vi "Autonomous Independent.vi"() -> ()   [LabVIEW 2016]
doc: "This VI is called when autonomous begins, and will automatically be terminated when autonomous ends. You can carry out timed or sensor driven robot movement independently without needing to return to the caller."
uses:
  <vilib>/Rock Robotics/WPI/ThirdParty/CanMotor/TalonSRX/WPI_CANTalonSRX_APIFeedbackSelect.ctl
  <vilib>/Rock Robotics/WPI/ThirdParty/CanMotor/TalonSRX/WPI_CANTalonSRX_Params.ctl
  <vilib>/Rock Robotics/WPI/ThirdParty/CanMotor/TalonSRX/WPI_CANTalonSRX_APIControlMode.ctl
  <vilib>/Rock Robotics/WPI/Utilities/WPI_GetSetVariantRefNum.vi
  <vilib>/Rock Robotics/Network Tables/NT Read String.vi
  <vilib>/Rock Robotics/Network Tables/NT Write Numeric Array.vi
  <vilib>/Rock Robotics/WPI/RobotDrive/WPI_RobotDriveArcadeDrive_Standard(NoSaturation).vi
  Robot Global Data.vi
panel:
  out "Distance":dbl
  out "RIGHT SIDE":dbl
  out "Encoder Position 4":dbl
  out "Encoder Position 3":dbl
  out "Encoder Position":dbl
  out "Encoder Position 2":dbl
  # "Be sure to right-click and choose Data Operations>>Make Current Value default if you want to save the array values with the VI"
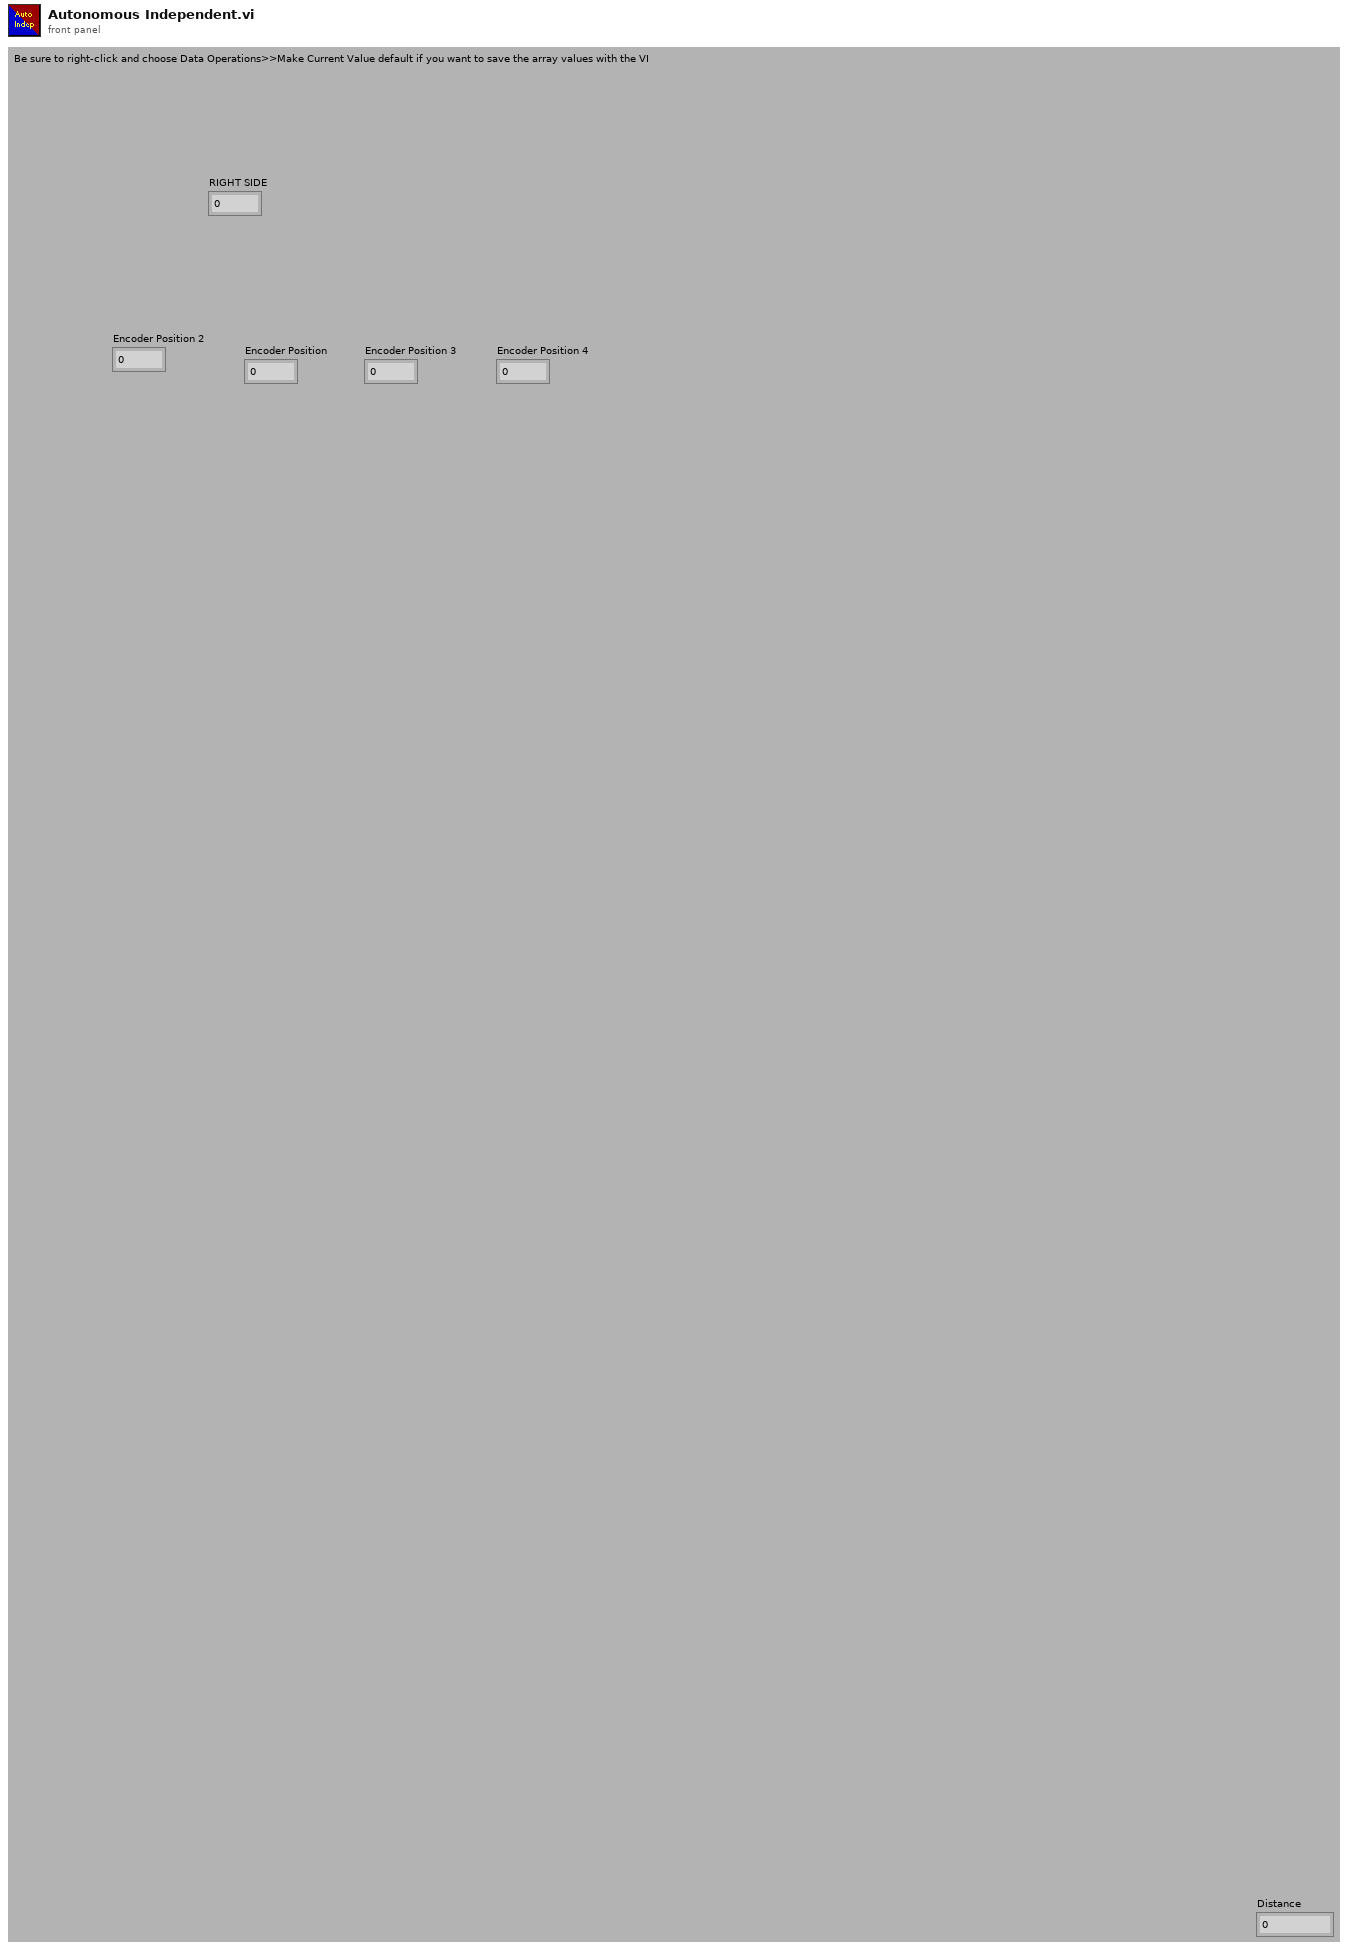
[diagram p1: front panel]
types:
  T1 = typedef "WPI_JoystickDevRef.ctl" = cluster{"Device":T2}
  T2 = typedef "WPI_JoystickDeviceEnum.ctl" = enum16{"USB 0", "USB 1", "USB 2", "USB 3", "USB 4", "USB 5"}
  T3 = typedef "WPI_EncoderDevRef.ctl" = cluster{"DevStatus":errorcluster, "EncoderIndex":T4, "CounterIndex":T5, "DistancePerCount":dbl, "Decoding Type":T6}
  T4 = typedef "FPGA_EncoderIdx.ctl" = enum8{"Enc 0", "Enc 1", "Enc 2", "Enc 3", "Enc 4", "Enc 5", "Enc 6", "Enc 7", "Invalid"}
  T5 = typedef "FPGA_CounterCtrSystemIndex.ctl" = enum8{"Ctr 0", "Ctr 1", "Ctr 2", "Ctr 3", "Ctr 4", "Ctr 5", "Ctr 6", "Ctr 7", "Invalid"}
  T6 = typedef "WPI_EncoderType.ctl" = enum16{"1x", "2x", "4x"}
  T7 = typedef "WPI_MotorControlDeviceRef.ctl" = cluster{"DeviceStatus":errorcluster, "Type":T8, "PWM":cluster{"PWM Channel":T9, "DeadBand":T10}, "CAN":cluster{"Device Number":u8, "SetOutput VI Ref":variant, "GetOutput VI Ref":variant, "Enable VI Ref":variant, "Disable VI Ref":variant, "Data":variant}, "Invert":bool}
  T8 = typedef "WPI_MotorControlType.ctl" = enum16{"PWM", "CAN"}
  T9 = typedef "FPGA_DIOPWMChannel.ctl" = enum8{"PWM 0", "PWM 1", "PWM 2", "PWM 3", "PWM 4", "PWM 5", "PWM 6", "PWM 7", "PWM 8", "PWM 9", "PWM MXP 0", "PWM MXP 1", "PWM MXP 2", "PWM MXP 3", "PWM MXP 4", "PWM MXP 5", "PWM MXP 6", "PWM MXP 7", "PWM MXP 8", "PWM MXP 9", "Invalid"}
  T10 = typedef "WPI_PWMDeadband.ctl" = cluster{"Name":string, "maxPositivePwm":i32, "minPositivePwm":i32, "centerPwm":i32, "maxNegativePwm":i32, "minNegativePwm":i32, "angularRange":u16}
  T11 = typedef "WPI_RobotDriveDevRef.ctl" = cluster{"DevStatus":errorcluster, "Motors[]":T7[], "Square Inputs":bool, "Max Output":dbl}
  T12 = typedef "WPI_CANTalonSRX_APIFeedbackSelect.ctl" = enum16{"Digital Quadrature Encoder", "Analog Potentiometer", "Analog Encoder", "Count on Quad-A (Rising-Edge)", "Count on Quad-A (Falling-Edge)", "CTR Magnetic Enc (Absolute)", "CTR Magnetic Enc (Relative)", "Pulse Width"}
  T13 = typedef "WPI_CANTalonSRX_APIControlMode.ctl" = enum8{"Percent VBus", "Speed", "Position", "Slave", "Unchanged / Invalid", "Voltage Compensation", "Current", "Motion Profile", "Motion Magic"}
  T14 = typedef "WPI_CANTalonSRX_Params.ctl" = u8
  T15 = typedef "WPI_CANTalonSRX_GlobalStatus.ctl" = cluster{"Applied Throttle":dbl, "Module Enabled":bool, "CAN Error":errorcluster, "Closed Loop Error":dbl, "Forward Limit Switch Closed":bool, "Reverse Limit Switch Closed":bool, "Sensor Position":dbl, "Sensor Velocity":dbl, "Current":dbl, "Sticky Fault - Over Temp":bool, "Sticky Fault - Under Voltage":bool, "Sticky Fault - Forward Limit":bool, "Sticky Fault - Reverse Limit":bool, "Sticky Fault - Forward Soft Limit":bool, "Sticky Fault - Reverse Soft Limit":bool, "Brake is Enabled":bool, "Encoder Position":dbl, "Encoder Velocity":dbl, "Encoder Index Count":dbl, "Encoder A Pin State":bool, "Encoder B Pin State":bool, "Encoder Index Pin State":bool, "Analog In":dbl, "Analog In Velocity":dbl, "Temperature (C)":dbl, "Battery Voltage":dbl, "Control 5 Is Supported":bool, "Current Profile Slot Select":dbl, "Pos Div 8":bool, "Vel Div 4":bool, "Pulse Width Position":i32, "Pulse Width Velocity":i32, "Pulse Width Rise To Rise (us)":i32, "Pulse Width Rise To Fall (us)":i32, "Mot Prof Active Is Under Run":bool, "Mot Prof Active Has Under Run":bool, "Mot Prof Active Is Last":bool, "Mot Prof Active Velocity Only":bool, "Mot Prof Active Is Valid":bool, "Mot Prof Buffer Is Full":bool, "Mot Prof Active Profile Slot Select":i32, "Mot Prof NextID":i32, "Mot Prof Count":i32, "Mot Prof Active Velocity":dbl, "Mot Prof Active Position":dbl, "Mot Prof Output Enable":i32, "UsageFrame":u32}
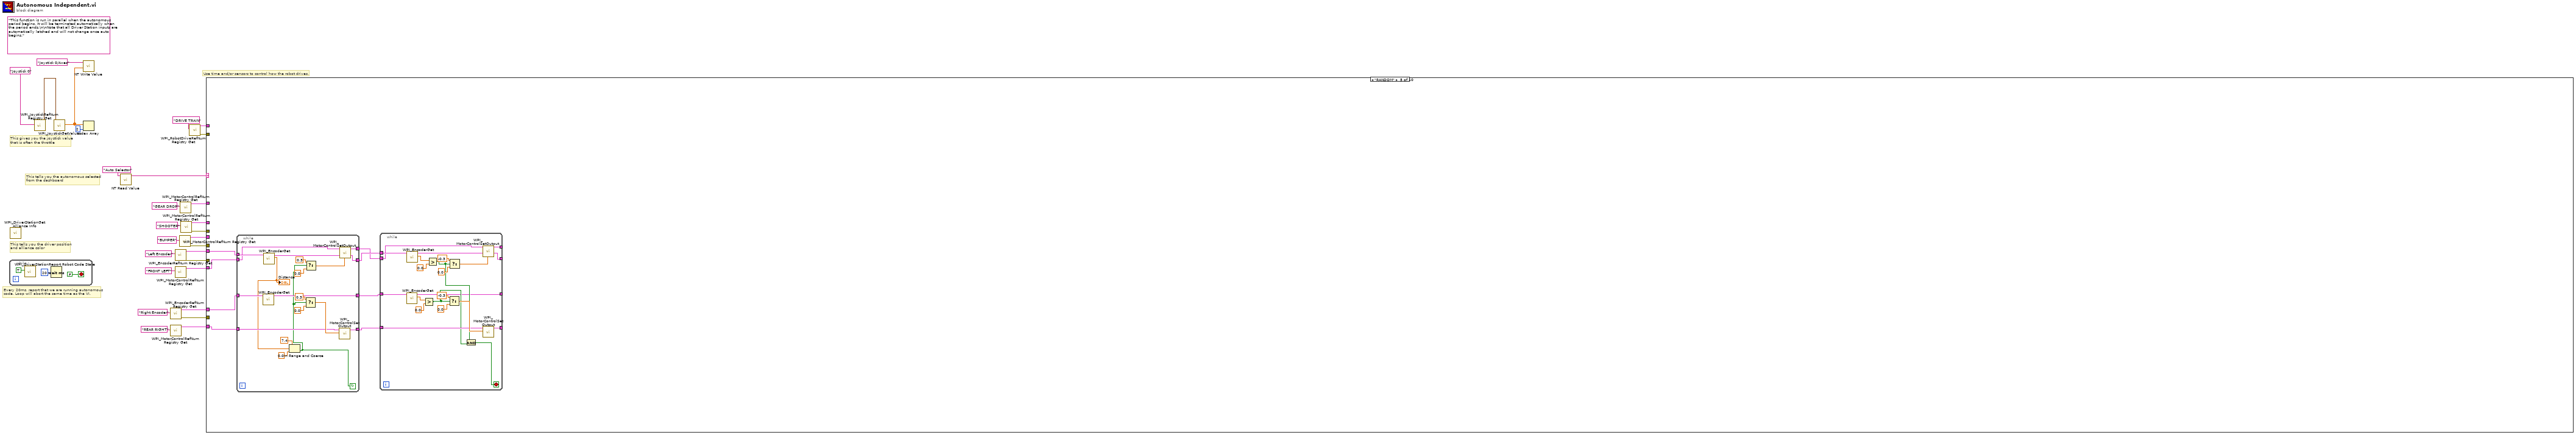
[diagram p0: block diagram]
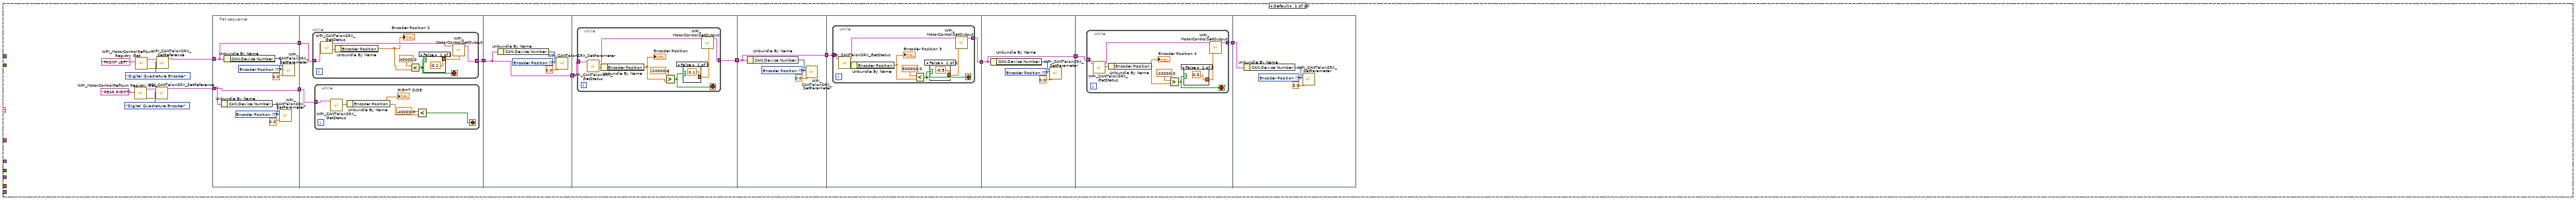
[diagram p2: hidden frame]
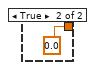
[diagram p3: hidden frame]
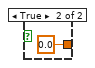
[diagram p4: hidden frame]
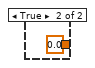
[diagram p5: hidden frame]
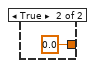
[diagram p6: hidden frame]
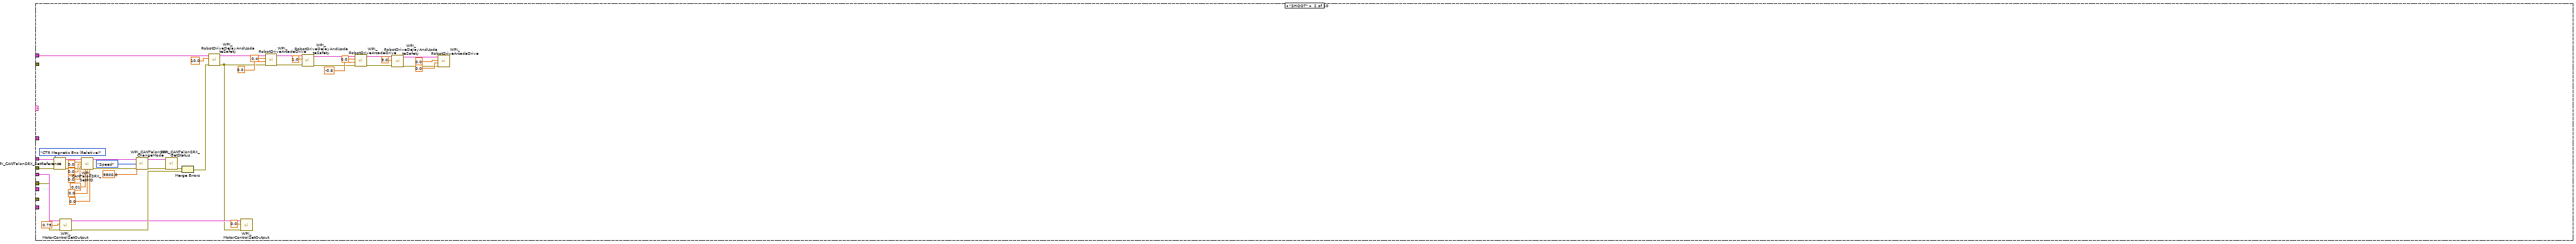
[diagram p7: hidden frame]
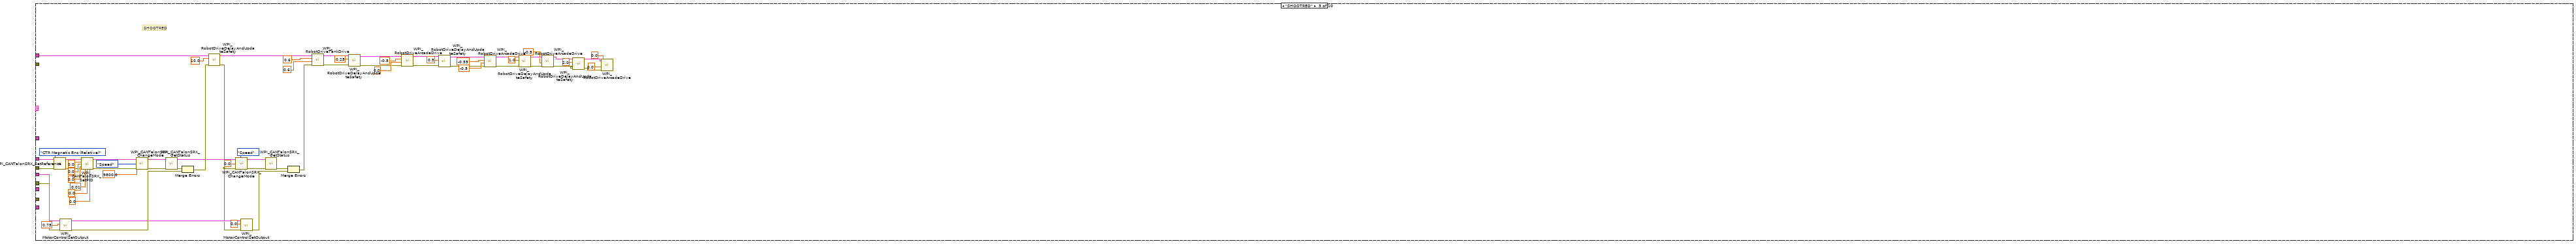
[diagram p8: hidden frame]
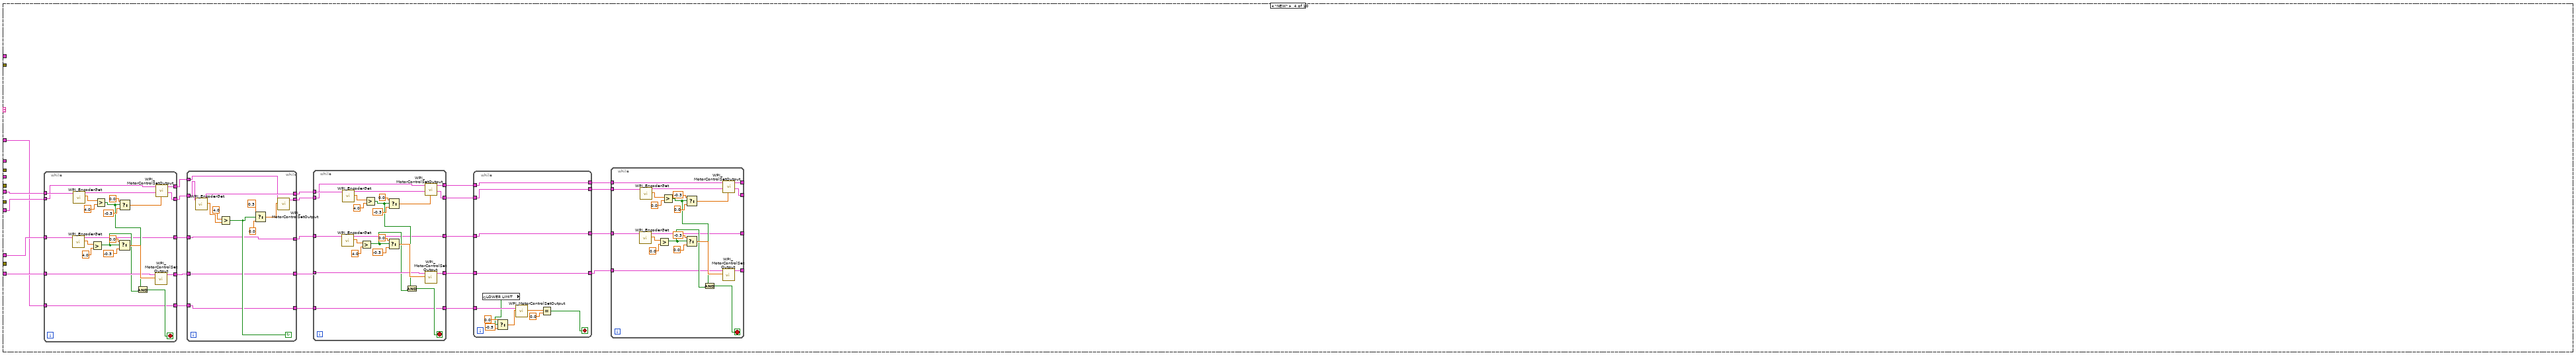
[diagram p9: hidden frame]
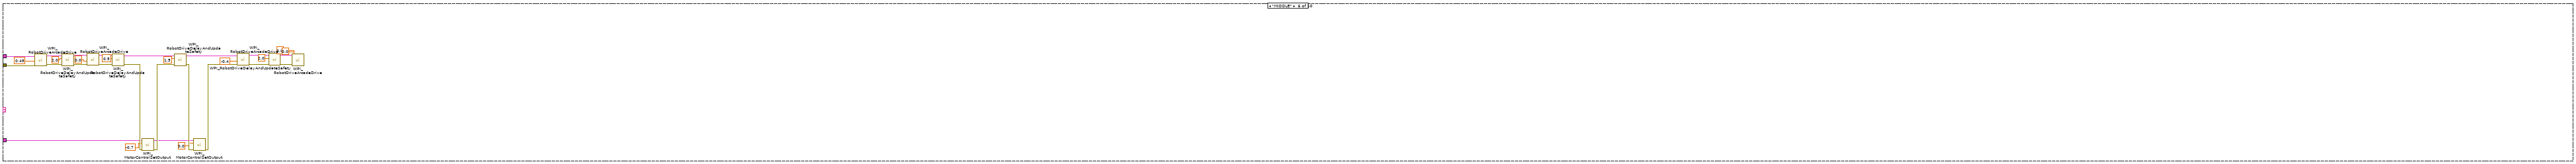
[diagram p10: hidden frame]
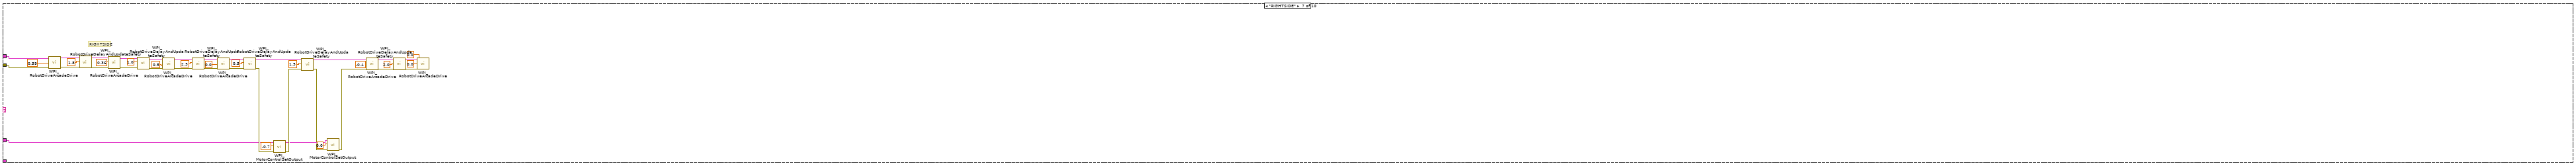
[diagram p11: hidden frame]
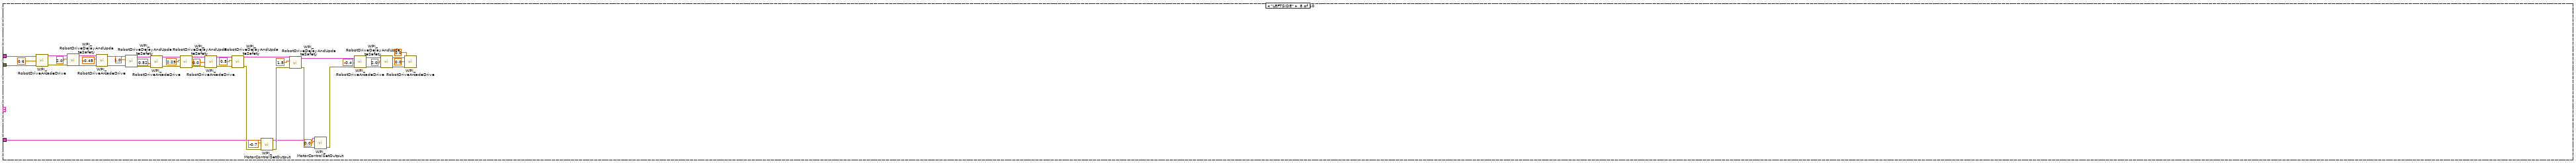
[diagram p12: hidden frame]
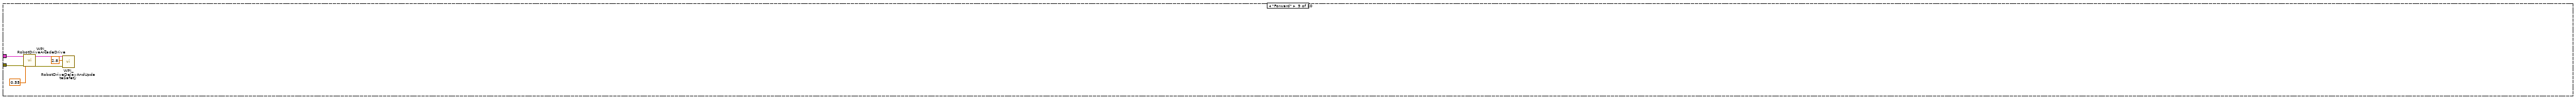
[diagram p13: hidden frame]
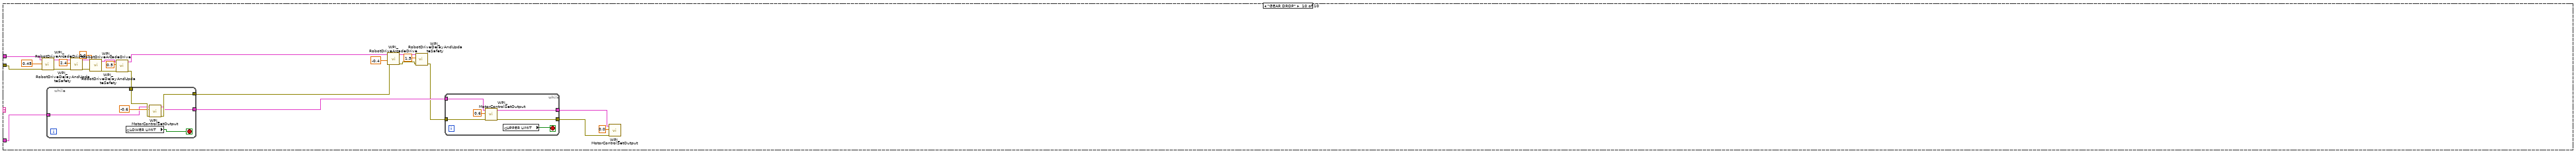
[diagram p14: hidden frame]
diagram:
  (unwired) "This function is run in parallel when the autonomous period begins. It will be terminated automatically when the period ends.\n\nNote that all Driver Station inputs are automatically latched and will not change once auto begins."
  # "Use time and/or sensors to control how the robot drives."
  # "This tells you the autonomous selected\nfrom the dashboard"
  # "Every 20ms, report that we are running autonomous\ncode. Loop will abort the same time as the VI."
  # "This gives you the joystick value\nthat is often the throttle"
  # "This tells you the driver position\nand alliance color"
  n1 = while {
    stop <- FALSE stop-if-true
    n2 = call <vilib>:"WPI_DriverStationReport Robot Code State.vi"("Autonomous"=TRUE) -> ()  [unwired: 10 in, 1 out]
    n3 = Wait (ms)(milliseconds to wait=u32 20) -> ()  [unwired: 1 out]
  }
  n4 = call <vilib>:"WPI_DriverStationGet Alliance Info.vi"() -> ()  [unwired: 12 out]
  n5 = call <vilib>:"WPI_JoystickRefNum Registry Get.vi"("refnum name"="Joystick 0") -> ("JoystickDevRef"=w27:T1)  [unwired: 1 in, 9 out]
  n6 = call <vilib>:"WPI_JoystickGetValues.vi"("JoystickDevRef"=w27) -> ("Axes"=w23:dbl[])  [unwired: 6 in, 4 out]
  n7 = call-poly <vilib>:"NT Write Value.vi"("Numeric Array"=w23, "Name"="Joystick 0/Axes") -> ()  [unwired: 9 in, 1 out]
  n8 = Index Array(array=w23, index=2) -> ()  [unwired: 1 out]
  n9 = call-poly <vilib>:"NT Read Value.vi"("Name"="Auto Selector") -> ("String"=w24:string)  [unwired: 9 in, 1 out]
  n10 = call <vilib>:"WPI_EncoderRefNum Registry Get.vi"("refnum name"="Right Encoder") -> ("error out"=w1:errorcluster, "EncoderDevRef"=w2:T3)  [unwired: 9 in]
  n11 = call <vilib>:"WPI_MotorControlRefNum Registry Get.vi"("refnum name"="REAR RIGHT") -> ("MotorControlDevRef"=w5:T7)  [unwired: 9 in, 1 out]
  n12 = call <vilib>:"WPI_EncoderRefNum Registry Get.vi"("refnum name"="Left Encoder") -> ("error out"=w3:errorcluster, "EncoderDevRef"=w4:T3)  [unwired: 9 in]
  n13 = call <vilib>:"WPI_MotorControlRefNum Registry Get.vi"("refnum name"="FRONT LEFT") -> ("MotorControlDevRef"=w8:T7)  [unwired: 9 in, 1 out]
  n14 = call <vilib>:"WPI_MotorControlRefNum Registry Get.vi"("refnum name"="BUMPER") -> ("error out"=w12:errorcluster, "MotorControlDevRef"=w13:T7)  [unwired: 9 in]
  n15 = call <vilib>:"WPI_MotorControlRefNum Registry Get.vi"("refnum name"="GEAR DROP") -> ("MotorControlDevRef"=w17:T7)  [unwired: 9 in, 1 out]
  n16 = call <vilib>:"WPI_MotorControlRefNum Registry Get.vi"("refnum name"="SHOOTER") -> ("error out"=w14:errorcluster, "MotorControlDevRef"=w15:T7)  [unwired: 9 in]
  n17 = call <vilib>:"WPI_RobotDriveRefNum Registry Get.vi"("refnum name"="DRIVE TRAIN") -> ("error out"=w19:errorcluster, "RobotDriveDevRef"=w20:T11)  [unwired: 9 in]
  n18 = case shown="\"RANDOM\"" w24 {
    tunnel: w20 -> [_ w155 w221 _ _ w431 w434 w517 w523 w548]
    tunnel: w19 -> [_ _ _ _ _ w430 w433 w516 w522 w547]
    tunnel: w17 -> [_ _ _ w247 _ w418 w432 w493 _ w528]
    tunnel: w15 -> [_ w161 w227 _ _ _ _ _ _ _]
    tunnel: w14 -> [_ w160 w226 _ _ _ _ _ _ _]
    tunnel: w13 -> [_ w146 w214 _ _ _ _ _ _ _]
    tunnel: w12 -> [_ w145 w213 _ _ _ _ _ _ _]
    tunnel: w4 -> [_ _ _ w261 w360 _ _ _ _ _]
    tunnel: w8 -> [_ _ _ w260 w361 _ _ _ _ _]
    tunnel: w5 -> [_ _ _ w258 w358 _ _ _ _ _]
    tunnel: w2 -> [_ _ _ w259 w359 _ _ _ _ _]
    tunnel: w3 -> [_ _ _ _ _ _ _ _ _ _]
    tunnel: w1 -> [_ _ _ _ _ _ _ _ _ _]
    frame Default {
      n19 = call <vilib>:"WPI_MotorControlRefNum Registry Get.vi"("refnum name"="REAR RIGHT") -> ("error out"=w36:errorcluster, "MotorControlDevRef"=w35:T7)  [unwired: 9 in]
      n20 = call <vilib>:"WPI_MotorControlRefNum Registry Get.vi"("refnum name"="FRONT LEFT") -> ("error out"=w48:errorcluster, "MotorControlDevRef"=w49:T7)  [unwired: 9 in]
      n21 = call <vilib>:"WPI_CANTalonSRX_SetReference.vi"("error in (no error)"=w36, "Feedback Reference"=WPI_CANTalonSRX_APIFeedbackSelect."Digital Quadrature Encoder", "CAN Talon SRX Ref"=w35) -> ("CAN Talon SRX Ref"=w33:T7)  [unwired: 7 in, 1 out]
      n22 = call <vilib>:"WPI_CANTalonSRX_SetReference.vi"("error in (no error)"=w48, "Feedback Reference"=WPI_CANTalonSRX_APIFeedbackSelect."Digital Quadrature Encoder", "CAN Talon SRX Ref"=w49) -> ("CAN Talon SRX Ref"=w44:T7)  [unwired: 7 in, 1 out]
      n23 = flat-sequence {
        tunnel: w44 -> [w55]
        tunnel: [w55] -> w43
        tunnel: w33 -> [w51]
        tunnel: [w51] -> w32
        tunnel: [w60] -> w46
        tunnel: w43 -> [w61]
        tunnel: w32 -> [w59]
        tunnel: w46 -> [w77]
        tunnel: [w77] -> w45
        tunnel: w45 -> [w82]
        tunnel: [w81] -> w42
        tunnel: w42 -> [w93]
        tunnel: [w93] -> w41
        tunnel: w41 -> [w98]
        tunnel: [w97] -> w40
        tunnel: w40 -> [w109]
        tunnel: [w109] -> w39
        tunnel: w39 -> [w114]
        tunnel: [w113] -> w38
        tunnel: w38 -> [w125]
        frame #0 {
          w53 = T14 77 items=["Slot 0 - P"=1, "Slot 0 - I"=2, "Slot 0 - D"=3, "Slot 0 - F"=4, "Slot 0 - I Zone"=5, "Slot 0 - Ramp Rate"=6, "Slot 1 - P"=11, "Slot 1 - I"=12, "Slot 1 - D"=13, "Slot 1 - F"=14, "Slot 1 - I Zone"=15, "Slot 1 - Ramp Rate"=16, "Soft Limit - Forward"=21, "Soft Limit - Reverse"=22, "Soft Limit - Forward Enable"=23, "Soft Limit - Reverse Enable"=24, "On Boot - Brake Mode"=31, "On Boot - Limit Normally Closed - Forward"=32, "On Boot - Limit Normally Closed - Reverse"=33, "On Boot - Limit Disabled - Forward"=34, "On Boot - Limit Disabled - Reverse"=35, "Fault - Over Temp"=41, "Fault - Under Voltage"=42, "Fault - Forward Limit"=43, "Fault - Reverse Limit"=44, "Fault - Hardware Failure"=45, "Fault - Forward Soft Limit"=46, "Fault - Reverse Soft Limit"=47, "Sticky Fault - Over Temp"=48, "Sticky Fault - Under Voltage"=49, "Sticky Fault - Forward Limit"=50, "Sticky Fault - Reverse Limit"=51, "Sticky Fault - Forward Soft Limit"=52, "Sticky Fault - Reverse Soft Limit"=53, "Applied Throttle"=61, "Closed-Loop Error"=62, "Select Feedback Device"=63, "Reverse Closed-Loop Output"=64, "Mode Select"=65, "Profile Slot Select"=66, "Ramp Throttle"=67, "Reverse Feedback Sensor"=68, "Limit Switch Enabled"=69, "Limit Switch Closed - Forward"=70, "Limit Switch Closed - Reverse"=71, "Sensor Position"=73, "Sensor Velocity"=74, "Current"=75, "Brake is Enabled"=76, "Encoder Position"=77, "Encoder Velocity"=78, "Encoder Index Rise Events"=79, "Encoder A Pin State"=80, "Encoder B Pin State"=81, "Encoder Index Pin State"=82, "Analog In with Overflow"=83, "Analog In Velocity"=84, "Temperature"=85, "Battery Voltage"=86, "Reset Count"=87, "Reset Flags"=88, "Firmware Version"=89, "Settings Changed"=90, "Quad Filter Enable"=91, "Ignore Disable Broadcast"=92, "I Accumulator"=93, "Status 1 Frame Rate Ms"=94, "Status 2 Frame Rate Ms"=95, "Status 3 Frame Rate Ms"=96, "Status 4 Frame Rate Ms"=97, "Status 6 Frame Rate Ms"=98, "Status 7 Frame Rate Ms"=99, "Enable Index Pin Clear Position"=100, "Peak Positive Output"=104, "Nominal Positive Output"=105, "Peak Negative Output"=106, "Nominal Negative Output"=107, "Quad Index Pin Polarity"=108, "Status 8 Frame Rate Ms"=109, "Allow Position Overflow"=110, "Slot 0 - Allowable Closed-Loop Error"=111, "Number Potentiometer Turns"=112, "Encoder Codes Per Rev"=113, "Pulse Width Decoded Position"=114, "Analog Position"=115, "Voltage Compensation Rate (V/s)"=116, "Slot 1 - Allowable Closed-Loop Error"=117, "Motion Profile Has Underrun Err"=119, "Reserved 120"=120, "Legacy Control Mode"=121, "Motion Magic Acceleration"=122, "Motion Magic Cruise Velocity"=123, "Status 10 Frame Rate"=124, "Current Limit Threshold"=125, "CustomParam0"=137, "CustomParam1"=138, "PersStorageSaving"=139, "ClearPositionOnLimitF"=144, "ClearPositionOnLimitR"=145, "NominalBatteryVoltage"=146, "SampleVelocityPeriod"=147, "SampleVelocityWindow"=148] ("Parameter")
          w57 = T14 77 items=["Slot 0 - P"=1, "Slot 0 - I"=2, "Slot 0 - D"=3, "Slot 0 - F"=4, "Slot 0 - I Zone"=5, "Slot 0 - Ramp Rate"=6, "Slot 1 - P"=11, "Slot 1 - I"=12, "Slot 1 - D"=13, "Slot 1 - F"=14, "Slot 1 - I Zone"=15, "Slot 1 - Ramp Rate"=16, "Soft Limit - Forward"=21, "Soft Limit - Reverse"=22, "Soft Limit - Forward Enable"=23, "Soft Limit - Reverse Enable"=24, "On Boot - Brake Mode"=31, "On Boot - Limit Normally Closed - Forward"=32, "On Boot - Limit Normally Closed - Reverse"=33, "On Boot - Limit Disabled - Forward"=34, "On Boot - Limit Disabled - Reverse"=35, "Fault - Over Temp"=41, "Fault - Under Voltage"=42, "Fault - Forward Limit"=43, "Fault - Reverse Limit"=44, "Fault - Hardware Failure"=45, "Fault - Forward Soft Limit"=46, "Fault - Reverse Soft Limit"=47, "Sticky Fault - Over Temp"=48, "Sticky Fault - Under Voltage"=49, "Sticky Fault - Forward Limit"=50, "Sticky Fault - Reverse Limit"=51, "Sticky Fault - Forward Soft Limit"=52, "Sticky Fault - Reverse Soft Limit"=53, "Applied Throttle"=61, "Closed-Loop Error"=62, "Select Feedback Device"=63, "Reverse Closed-Loop Output"=64, "Mode Select"=65, "Profile Slot Select"=66, "Ramp Throttle"=67, "Reverse Feedback Sensor"=68, "Limit Switch Enabled"=69, "Limit Switch Closed - Forward"=70, "Limit Switch Closed - Reverse"=71, "Sensor Position"=73, "Sensor Velocity"=74, "Current"=75, "Brake is Enabled"=76, "Encoder Position"=77, "Encoder Velocity"=78, "Encoder Index Rise Events"=79, "Encoder A Pin State"=80, "Encoder B Pin State"=81, "Encoder Index Pin State"=82, "Analog In with Overflow"=83, "Analog In Velocity"=84, "Temperature"=85, "Battery Voltage"=86, "Reset Count"=87, "Reset Flags"=88, "Firmware Version"=89, "Settings Changed"=90, "Quad Filter Enable"=91, "Ignore Disable Broadcast"=92, "I Accumulator"=93, "Status 1 Frame Rate Ms"=94, "Status 2 Frame Rate Ms"=95, "Status 3 Frame Rate Ms"=96, "Status 4 Frame Rate Ms"=97, "Status 6 Frame Rate Ms"=98, "Status 7 Frame Rate Ms"=99, "Enable Index Pin Clear Position"=100, "Peak Positive Output"=104, "Nominal Positive Output"=105, "Peak Negative Output"=106, "Nominal Negative Output"=107, "Quad Index Pin Polarity"=108, "Status 8 Frame Rate Ms"=109, "Allow Position Overflow"=110, "Slot 0 - Allowable Closed-Loop Error"=111, "Number Potentiometer Turns"=112, "Encoder Codes Per Rev"=113, "Pulse Width Decoded Position"=114, "Analog Position"=115, "Voltage Compensation Rate (V/s)"=116, "Slot 1 - Allowable Closed-Loop Error"=117, "Motion Profile Has Underrun Err"=119, "Reserved 120"=120, "Legacy Control Mode"=121, "Motion Magic Acceleration"=122, "Motion Magic Cruise Velocity"=123, "Status 10 Frame Rate"=124, "Current Limit Threshold"=125, "CustomParam0"=137, "CustomParam1"=138, "PersStorageSaving"=139, "ClearPositionOnLimitF"=144, "ClearPositionOnLimitR"=145, "NominalBatteryVoltage"=146, "SampleVelocityPeriod"=147, "SampleVelocityWindow"=148] ("Parameter")
          n24 = Unbundle By Name(w51) -> ("CAN.Device Number"=w52:u8)
          n25 = Unbundle By Name(w55) -> ("CAN.Device Number"=w58:u8)
          n26 = call <vilib>:"WPI_CANTalonSRX_SetParameter.vi"("Value"=0.0, "Parameter"=w53, "Device ID (0)"=w52) -> ()  [unwired: 7 in, 2 out]
          n27 = call <vilib>:"WPI_CANTalonSRX_SetParameter.vi"("Value"=0.0, "Parameter"=w57, "Device ID (0)"=w58) -> ()  [unwired: 7 in, 2 out]
        }
        frame #1 {
          n28 = while {
            tunnel: w61 -> [w68]
            tunnel: [w67] -> w60
            stop <- w71 stop-if-true
            n29 = call <vilib>:"WPI_CANTalonSRX_GetStatus.vi"("CAN Talon SRX Ref"=w68) -> ("Talon SRX Status"=w74:T15, "CAN Talon SRX Ref"=w73:T7)  [unwired: 8 in, 1 out]
            n30 = Unbundle By Name(w74) -> ("Encoder Position"=w70:dbl)
            "Encoder Position 2" <- w70
            n31 = Less?(x=40000.0, y=w70) -> (x < y?=w71:bool)
            n32 = case shown="False" w71 {
              tunnel: [-0.1 ("x") 0.0 ("x")] -> w72
              frame False {
              }
              frame True {
              }
            }
            n33 = call <vilib>:"WPI_MotorControlSetOutput.vi"("Output"=w72, "MotorControlDevRef"=w73) -> ("MotorControlDevRef"=w67:T7)  [unwired: 7 in, 2 out]
          }
          n34 = while {
            tunnel: w59 -> [w66]
            stop <- w63 stop-if-true
            n35 = call <vilib>:"WPI_CANTalonSRX_GetStatus.vi"("CAN Talon SRX Ref"=w66) -> ("Talon SRX Status"=w62:T15)  [unwired: 8 in, 2 out]
            n36 = Unbundle By Name(w62) -> ("Encoder Position"=w65:dbl)
            "RIGHT SIDE" <- w65
            n37 = Less?(x=-40000.0, y=w65) -> (x < y?=w63:bool)
          }
        }
        frame #2 {
          w79 = T14 77 items=["Slot 0 - P"=1, "Slot 0 - I"=2, "Slot 0 - D"=3, "Slot 0 - F"=4, "Slot 0 - I Zone"=5, "Slot 0 - Ramp Rate"=6, "Slot 1 - P"=11, "Slot 1 - I"=12, "Slot 1 - D"=13, "Slot 1 - F"=14, "Slot 1 - I Zone"=15, "Slot 1 - Ramp Rate"=16, "Soft Limit - Forward"=21, "Soft Limit - Reverse"=22, "Soft Limit - Forward Enable"=23, "Soft Limit - Reverse Enable"=24, "On Boot - Brake Mode"=31, "On Boot - Limit Normally Closed - Forward"=32, "On Boot - Limit Normally Closed - Reverse"=33, "On Boot - Limit Disabled - Forward"=34, "On Boot - Limit Disabled - Reverse"=35, "Fault - Over Temp"=41, "Fault - Under Voltage"=42, "Fault - Forward Limit"=43, "Fault - Reverse Limit"=44, "Fault - Hardware Failure"=45, "Fault - Forward Soft Limit"=46, "Fault - Reverse Soft Limit"=47, "Sticky Fault - Over Temp"=48, "Sticky Fault - Under Voltage"=49, "Sticky Fault - Forward Limit"=50, "Sticky Fault - Reverse Limit"=51, "Sticky Fault - Forward Soft Limit"=52, "Sticky Fault - Reverse Soft Limit"=53, "Applied Throttle"=61, "Closed-Loop Error"=62, "Select Feedback Device"=63, "Reverse Closed-Loop Output"=64, "Mode Select"=65, "Profile Slot Select"=66, "Ramp Throttle"=67, "Reverse Feedback Sensor"=68, "Limit Switch Enabled"=69, "Limit Switch Closed - Forward"=70, "Limit Switch Closed - Reverse"=71, "Sensor Position"=73, "Sensor Velocity"=74, "Current"=75, "Brake is Enabled"=76, "Encoder Position"=77, "Encoder Velocity"=78, "Encoder Index Rise Events"=79, "Encoder A Pin State"=80, "Encoder B Pin State"=81, "Encoder Index Pin State"=82, "Analog In with Overflow"=83, "Analog In Velocity"=84, "Temperature"=85, "Battery Voltage"=86, "Reset Count"=87, "Reset Flags"=88, "Firmware Version"=89, "Settings Changed"=90, "Quad Filter Enable"=91, "Ignore Disable Broadcast"=92, "I Accumulator"=93, "Status 1 Frame Rate Ms"=94, "Status 2 Frame Rate Ms"=95, "Status 3 Frame Rate Ms"=96, "Status 4 Frame Rate Ms"=97, "Status 6 Frame Rate Ms"=98, "Status 7 Frame Rate Ms"=99, "Enable Index Pin Clear Position"=100, "Peak Positive Output"=104, "Nominal Positive Output"=105, "Peak Negative Output"=106, "Nominal Negative Output"=107, "Quad Index Pin Polarity"=108, "Status 8 Frame Rate Ms"=109, "Allow Position Overflow"=110, "Slot 0 - Allowable Closed-Loop Error"=111, "Number Potentiometer Turns"=112, "Encoder Codes Per Rev"=113, "Pulse Width Decoded Position"=114, "Analog Position"=115, "Voltage Compensation Rate (V/s)"=116, "Slot 1 - Allowable Closed-Loop Error"=117, "Motion Profile Has Underrun Err"=119, "Reserved 120"=120, "Legacy Control Mode"=121, "Motion Magic Acceleration"=122, "Motion Magic Cruise Velocity"=123, "Status 10 Frame Rate"=124, "Current Limit Threshold"=125, "CustomParam0"=137, "CustomParam1"=138, "PersStorageSaving"=139, "ClearPositionOnLimitF"=144, "ClearPositionOnLimitR"=145, "NominalBatteryVoltage"=146, "SampleVelocityPeriod"=147, "SampleVelocityWindow"=148] ("Parameter")
          n38 = Unbundle By Name(w77) -> ("CAN.Device Number"=w80:u8)
          n39 = call <vilib>:"WPI_CANTalonSRX_SetParameter.vi"("Value"=0.0, "Parameter"=w79, "Device ID (0)"=w80) -> ()  [unwired: 7 in, 2 out]
        }
        frame #3 {
          n40 = while {
            tunnel: w82 -> [w84]
            tunnel: [w83] -> w81
            stop <- w87 stop-if-true
            n41 = call <vilib>:"WPI_CANTalonSRX_GetStatus.vi"("CAN Talon SRX Ref"=w84) -> ("Talon SRX Status"=w90:T15, "CAN Talon SRX Ref"=w89:T7)  [unwired: 8 in, 1 out]
            n42 = Unbundle By Name(w90) -> ("Encoder Position"=w86:dbl)
            "Encoder Position" <- w86
            n43 = Greater?(x=-20000.0 ("y"), y=w86) -> (0:w87:bool)
            n44 = case shown="False" w87 {
              tunnel: [0.1 ("x") 0.0 ("x")] -> w88
              frame False {
              }
              frame True {
              }
            }
            n45 = call <vilib>:"WPI_MotorControlSetOutput.vi"("Output"=w88, "MotorControlDevRef"=w89) -> ("MotorControlDevRef"=w83:T7)  [unwired: 7 in, 2 out]
          }
        }
        frame #4 {
          w95 = T14 77 items=["Slot 0 - P"=1, "Slot 0 - I"=2, "Slot 0 - D"=3, "Slot 0 - F"=4, "Slot 0 - I Zone"=5, "Slot 0 - Ramp Rate"=6, "Slot 1 - P"=11, "Slot 1 - I"=12, "Slot 1 - D"=13, "Slot 1 - F"=14, "Slot 1 - I Zone"=15, "Slot 1 - Ramp Rate"=16, "Soft Limit - Forward"=21, "Soft Limit - Reverse"=22, "Soft Limit - Forward Enable"=23, "Soft Limit - Reverse Enable"=24, "On Boot - Brake Mode"=31, "On Boot - Limit Normally Closed - Forward"=32, "On Boot - Limit Normally Closed - Reverse"=33, "On Boot - Limit Disabled - Forward"=34, "On Boot - Limit Disabled - Reverse"=35, "Fault - Over Temp"=41, "Fault - Under Voltage"=42, "Fault - Forward Limit"=43, "Fault - Reverse Limit"=44, "Fault - Hardware Failure"=45, "Fault - Forward Soft Limit"=46, "Fault - Reverse Soft Limit"=47, "Sticky Fault - Over Temp"=48, "Sticky Fault - Under Voltage"=49, "Sticky Fault - Forward Limit"=50, "Sticky Fault - Reverse Limit"=51, "Sticky Fault - Forward Soft Limit"=52, "Sticky Fault - Reverse Soft Limit"=53, "Applied Throttle"=61, "Closed-Loop Error"=62, "Select Feedback Device"=63, "Reverse Closed-Loop Output"=64, "Mode Select"=65, "Profile Slot Select"=66, "Ramp Throttle"=67, "Reverse Feedback Sensor"=68, "Limit Switch Enabled"=69, "Limit Switch Closed - Forward"=70, "Limit Switch Closed - Reverse"=71, "Sensor Position"=73, "Sensor Velocity"=74, "Current"=75, "Brake is Enabled"=76, "Encoder Position"=77, "Encoder Velocity"=78, "Encoder Index Rise Events"=79, "Encoder A Pin State"=80, "Encoder B Pin State"=81, "Encoder Index Pin State"=82, "Analog In with Overflow"=83, "Analog In Velocity"=84, "Temperature"=85, "Battery Voltage"=86, "Reset Count"=87, "Reset Flags"=88, "Firmware Version"=89, "Settings Changed"=90, "Quad Filter Enable"=91, "Ignore Disable Broadcast"=92, "I Accumulator"=93, "Status 1 Frame Rate Ms"=94, "Status 2 Frame Rate Ms"=95, "Status 3 Frame Rate Ms"=96, "Status 4 Frame Rate Ms"=97, "Status 6 Frame Rate Ms"=98, "Status 7 Frame Rate Ms"=99, "Enable Index Pin Clear Position"=100, "Peak Positive Output"=104, "Nominal Positive Output"=105, "Peak Negative Output"=106, "Nominal Negative Output"=107, "Quad Index Pin Polarity"=108, "Status 8 Frame Rate Ms"=109, "Allow Position Overflow"=110, "Slot 0 - Allowable Closed-Loop Error"=111, "Number Potentiometer Turns"=112, "Encoder Codes Per Rev"=113, "Pulse Width Decoded Position"=114, "Analog Position"=115, "Voltage Compensation Rate (V/s)"=116, "Slot 1 - Allowable Closed-Loop Error"=117, "Motion Profile Has Underrun Err"=119, "Reserved 120"=120, "Legacy Control Mode"=121, "Motion Magic Acceleration"=122, "Motion Magic Cruise Velocity"=123, "Status 10 Frame Rate"=124, "Current Limit Threshold"=125, "CustomParam0"=137, "CustomParam1"=138, "PersStorageSaving"=139, "ClearPositionOnLimitF"=144, "ClearPositionOnLimitR"=145, "NominalBatteryVoltage"=146, "SampleVelocityPeriod"=147, "SampleVelocityWindow"=148] ("Parameter")
          n46 = Unbundle By Name(w93) -> ("CAN.Device Number"=w96:u8)
          n47 = call <vilib>:"WPI_CANTalonSRX_SetParameter.vi"("Value"=0.0, "Parameter"=w95, "Device ID (0)"=w96) -> ()  [unwired: 7 in, 2 out]
        }
        frame #5 {
          n48 = while {
            tunnel: w98 -> [w100]
            tunnel: [w99] -> w97
            stop <- w103 stop-if-true
            n49 = call <vilib>:"WPI_CANTalonSRX_GetStatus.vi"("CAN Talon SRX Ref"=w100) -> ("Talon SRX Status"=w106:T15, "CAN Talon SRX Ref"=w105:T7)  [unwired: 8 in, 1 out]
            n50 = Unbundle By Name(w106) -> ("Encoder Position"=w102:dbl)
            "Encoder Position 3" <- w102
            n51 = Less?(x=500000.0, y=w102) -> (x < y?=w103:bool)
            n52 = case shown="False" w103 {
              tunnel: [-0.5 ("x") 0.0 ("x")] -> w104
              frame False {
              }
              frame True {
              }
            }
            n53 = call <vilib>:"WPI_MotorControlSetOutput.vi"("Output"=w104, "MotorControlDevRef"=w105) -> ("MotorControlDevRef"=w99:T7)  [unwired: 7 in, 2 out]
          }
        }
        frame #6 {
          w111 = T14 77 items=["Slot 0 - P"=1, "Slot 0 - I"=2, "Slot 0 - D"=3, "Slot 0 - F"=4, "Slot 0 - I Zone"=5, "Slot 0 - Ramp Rate"=6, "Slot 1 - P"=11, "Slot 1 - I"=12, "Slot 1 - D"=13, "Slot 1 - F"=14, "Slot 1 - I Zone"=15, "Slot 1 - Ramp Rate"=16, "Soft Limit - Forward"=21, "Soft Limit - Reverse"=22, "Soft Limit - Forward Enable"=23, "Soft Limit - Reverse Enable"=24, "On Boot - Brake Mode"=31, "On Boot - Limit Normally Closed - Forward"=32, "On Boot - Limit Normally Closed - Reverse"=33, "On Boot - Limit Disabled - Forward"=34, "On Boot - Limit Disabled - Reverse"=35, "Fault - Over Temp"=41, "Fault - Under Voltage"=42, "Fault - Forward Limit"=43, "Fault - Reverse Limit"=44, "Fault - Hardware Failure"=45, "Fault - Forward Soft Limit"=46, "Fault - Reverse Soft Limit"=47, "Sticky Fault - Over Temp"=48, "Sticky Fault - Under Voltage"=49, "Sticky Fault - Forward Limit"=50, "Sticky Fault - Reverse Limit"=51, "Sticky Fault - Forward Soft Limit"=52, "Sticky Fault - Reverse Soft Limit"=53, "Applied Throttle"=61, "Closed-Loop Error"=62, "Select Feedback Device"=63, "Reverse Closed-Loop Output"=64, "Mode Select"=65, "Profile Slot Select"=66, "Ramp Throttle"=67, "Reverse Feedback Sensor"=68, "Limit Switch Enabled"=69, "Limit Switch Closed - Forward"=70, "Limit Switch Closed - Reverse"=71, "Sensor Position"=73, "Sensor Velocity"=74, "Current"=75, "Brake is Enabled"=76, "Encoder Position"=77, "Encoder Velocity"=78, "Encoder Index Rise Events"=79, "Encoder A Pin State"=80, "Encoder B Pin State"=81, "Encoder Index Pin State"=82, "Analog In with Overflow"=83, "Analog In Velocity"=84, "Temperature"=85, "Battery Voltage"=86, "Reset Count"=87, "Reset Flags"=88, "Firmware Version"=89, "Settings Changed"=90, "Quad Filter Enable"=91, "Ignore Disable Broadcast"=92, "I Accumulator"=93, "Status 1 Frame Rate Ms"=94, "Status 2 Frame Rate Ms"=95, "Status 3 Frame Rate Ms"=96, "Status 4 Frame Rate Ms"=97, "Status 6 Frame Rate Ms"=98, "Status 7 Frame Rate Ms"=99, "Enable Index Pin Clear Position"=100, "Peak Positive Output"=104, "Nominal Positive Output"=105, "Peak Negative Output"=106, "Nominal Negative Output"=107, "Quad Index Pin Polarity"=108, "Status 8 Frame Rate Ms"=109, "Allow Position Overflow"=110, "Slot 0 - Allowable Closed-Loop Error"=111, "Number Potentiometer Turns"=112, "Encoder Codes Per Rev"=113, "Pulse Width Decoded Position"=114, "Analog Position"=115, "Voltage Compensation Rate (V/s)"=116, "Slot 1 - Allowable Closed-Loop Error"=117, "Motion Profile Has Underrun Err"=119, "Reserved 120"=120, "Legacy Control Mode"=121, "Motion Magic Acceleration"=122, "Motion Magic Cruise Velocity"=123, "Status 10 Frame Rate"=124, "Current Limit Threshold"=125, "CustomParam0"=137, "CustomParam1"=138, "PersStorageSaving"=139, "ClearPositionOnLimitF"=144, "ClearPositionOnLimitR"=145, "NominalBatteryVoltage"=146, "SampleVelocityPeriod"=147, "SampleVelocityWindow"=148] ("Parameter")
          n54 = Unbundle By Name(w109) -> ("CAN.Device Number"=w110:u8)
          n55 = call <vilib>:"WPI_CANTalonSRX_SetParameter.vi"("Value"=0.0, "Parameter"=w111, "Device ID (0)"=w110) -> ()  [unwired: 7 in, 2 out]
        }
        frame #7 {
          n56 = while {
            tunnel: w114 -> [w116]
            tunnel: [w115] -> w113
            stop <- w119 stop-if-true
            n57 = call <vilib>:"WPI_CANTalonSRX_GetStatus.vi"("CAN Talon SRX Ref"=w116) -> ("Talon SRX Status"=w122:T15, "CAN Talon SRX Ref"=w121:T7)  [unwired: 8 in, 1 out]
            n58 = Unbundle By Name(w122) -> ("Encoder Position"=w118:dbl)
            "Encoder Position 4" <- w118
            n59 = Greater?(x=-20000.0, y=w118) -> (0:w119:bool)
            n60 = case shown="False" w119 {
              tunnel: [0.3 ("x") 0.0 ("x")] -> w120
              frame False {
              }
              frame True {
              }
            }
            n61 = call <vilib>:"WPI_MotorControlSetOutput.vi"("Output"=w120, "MotorControlDevRef"=w121) -> ("MotorControlDevRef"=w115:T7)  [unwired: 7 in, 2 out]
          }
        }
        frame #8 {
          w127 = T14 77 items=["Slot 0 - P"=1, "Slot 0 - I"=2, "Slot 0 - D"=3, "Slot 0 - F"=4, "Slot 0 - I Zone"=5, "Slot 0 - Ramp Rate"=6, "Slot 1 - P"=11, "Slot 1 - I"=12, "Slot 1 - D"=13, "Slot 1 - F"=14, "Slot 1 - I Zone"=15, "Slot 1 - Ramp Rate"=16, "Soft Limit - Forward"=21, "Soft Limit - Reverse"=22, "Soft Limit - Forward Enable"=23, "Soft Limit - Reverse Enable"=24, "On Boot - Brake Mode"=31, "On Boot - Limit Normally Closed - Forward"=32, "On Boot - Limit Normally Closed - Reverse"=33, "On Boot - Limit Disabled - Forward"=34, "On Boot - Limit Disabled - Reverse"=35, "Fault - Over Temp"=41, "Fault - Under Voltage"=42, "Fault - Forward Limit"=43, "Fault - Reverse Limit"=44, "Fault - Hardware Failure"=45, "Fault - Forward Soft Limit"=46, "Fault - Reverse Soft Limit"=47, "Sticky Fault - Over Temp"=48, "Sticky Fault - Under Voltage"=49, "Sticky Fault - Forward Limit"=50, "Sticky Fault - Reverse Limit"=51, "Sticky Fault - Forward Soft Limit"=52, "Sticky Fault - Reverse Soft Limit"=53, "Applied Throttle"=61, "Closed-Loop Error"=62, "Select Feedback Device"=63, "Reverse Closed-Loop Output"=64, "Mode Select"=65, "Profile Slot Select"=66, "Ramp Throttle"=67, "Reverse Feedback Sensor"=68, "Limit Switch Enabled"=69, "Limit Switch Closed - Forward"=70, "Limit Switch Closed - Reverse"=71, "Sensor Position"=73, "Sensor Velocity"=74, "Current"=75, "Brake is Enabled"=76, "Encoder Position"=77, "Encoder Velocity"=78, "Encoder Index Rise Events"=79, "Encoder A Pin State"=80, "Encoder B Pin State"=81, "Encoder Index Pin State"=82, "Analog In with Overflow"=83, "Analog In Velocity"=84, "Temperature"=85, "Battery Voltage"=86, "Reset Count"=87, "Reset Flags"=88, "Firmware Version"=89, "Settings Changed"=90, "Quad Filter Enable"=91, "Ignore Disable Broadcast"=92, "I Accumulator"=93, "Status 1 Frame Rate Ms"=94, "Status 2 Frame Rate Ms"=95, "Status 3 Frame Rate Ms"=96, "Status 4 Frame Rate Ms"=97, "Status 6 Frame Rate Ms"=98, "Status 7 Frame Rate Ms"=99, "Enable Index Pin Clear Position"=100, "Peak Positive Output"=104, "Nominal Positive Output"=105, "Peak Negative Output"=106, "Nominal Negative Output"=107, "Quad Index Pin Polarity"=108, "Status 8 Frame Rate Ms"=109, "Allow Position Overflow"=110, "Slot 0 - Allowable Closed-Loop Error"=111, "Number Potentiometer Turns"=112, "Encoder Codes Per Rev"=113, "Pulse Width Decoded Position"=114, "Analog Position"=115, "Voltage Compensation Rate (V/s)"=116, "Slot 1 - Allowable Closed-Loop Error"=117, "Motion Profile Has Underrun Err"=119, "Reserved 120"=120, "Legacy Control Mode"=121, "Motion Magic Acceleration"=122, "Motion Magic Cruise Velocity"=123, "Status 10 Frame Rate"=124, "Current Limit Threshold"=125, "CustomParam0"=137, "CustomParam1"=138, "PersStorageSaving"=139, "ClearPositionOnLimitF"=144, "ClearPositionOnLimitR"=145, "NominalBatteryVoltage"=146, "SampleVelocityPeriod"=147, "SampleVelocityWindow"=148] ("Parameter")
          n62 = Unbundle By Name(w125) -> ("CAN.Device Number"=w126:u8)
          n63 = call <vilib>:"WPI_CANTalonSRX_SetParameter.vi"("Value"=0.0, "Parameter"=w127, "Device ID (0)"=w126) -> ()  [unwired: 7 in, 2 out]
        }
      }
    }
    frame "SHOOT" {
      n64 = call <vilib>:"WPI_CANTalonSRX_SetReference.vi"("error in (no error)"=w160, "Feedback Reference"=WPI_CANTalonSRX_APIFeedbackSelect."CTR Magnetic Enc (Relative)", "CAN Talon SRX Ref"=w161) -> ("error out"=w159:errorcluster, "CAN Talon SRX Ref"=w169:T7)  [unwired: 7 in]
      n65 = call <vilib>:"WPI_MotorControlSetOutput.vi"("error in (no error)"=w145, "Output"=0.75, "MotorControlDevRef"=w146) -> ("error out"=w142:errorcluster, "MotorControlDevRef"=w140:T7)  [unwired: 6 in, 1 out]
      n66 = call <vilib>:"WPI_CANTalonSRX_SetPID.vi"("CAN Talon SRX Ref"=w169, "P"=0.0, "I"=0.0, "D"=0.0, "error in (no error)"=w159, "F"=0.01, "I Zone"=0.0, "Ramp Rate"=0.0) -> ("CAN Talon SRX Ref"=w166:T7, "error out"=w158:errorcluster)  [unwired: 6 in]
      n67 = call <vilib>:"WPI_CANTalonSRX_ChangeMode.vi"("error in (no error)"=w158, "Output"=9800.0 ("y"), "Control Mode"=WPI_CANTalonSRX_APIControlMode."Speed", "CAN Talon SRX Ref"=w166) -> ("error out"=w157:errorcluster, "CAN Talon SRX Ref"=w162:T7)  [unwired: 6 in]
      n68 = call <vilib>:"WPI_CANTalonSRX_GetStatus.vi"("error in (no error)"=w157, "CAN Talon SRX Ref"=w162) -> ("error out"=w143:errorcluster)  [unwired: 7 in, 2 out]
      n69 = Merge Errors(w143, w142) -> (w141:errorcluster)
      n70 = call <vilib>:"WPI_RobotDriveDelayAndUpdateSafety.vi"("error in (no error)"=w141, "Delay (s)"=10.0, "RobotDriveDevRef"=w155) -> ("error out"=w139:errorcluster, "RobotDriveDevRef 2"=w156:T11)  [unwired: 7 in]
      n71 = call <vilib>:"WPI_MotorControlSetOutput.vi"("error in (no error)"=w139, "Output"=0.0, "MotorControlDevRef"=w140) -> ()  [unwired: 6 in, 3 out]
      n72 = call-poly <vilib>:"WPI_RobotDriveArcadeDrive.vi"("error in (no error)"=w139, "Y axis value"=0.0, "X axis value"=0.4, "RobotDriveDevRef"=w156) -> ("error out"=w152:errorcluster, "RobotDriveDevRef"=w153:T11)  [unwired: 5 in, 1 out]
      n73 = call <vilib>:"WPI_RobotDriveDelayAndUpdateSafety.vi"("error in (no error)"=w152, "Delay (s)"=1.0, "RobotDriveDevRef"=w153) -> ("error out"=w132:errorcluster, "RobotDriveDevRef 2"=w131:T11)  [unwired: 7 in]
      n74 = call-poly <vilib>:"WPI_RobotDriveArcadeDrive.vi"("error in (no error)"=w132, "Y axis value"=-0.6, "X axis value"=0.0, "RobotDriveDevRef"=w131) -> ("error out"=w135:errorcluster, "RobotDriveDevRef"=w136:T11)  [unwired: 5 in, 1 out]
      n75 = call <vilib>:"WPI_RobotDriveDelayAndUpdateSafety.vi"("error in (no error)"=w135, "Delay (s)"=3.0, "RobotDriveDevRef"=w136) -> ("error out"=w129:errorcluster, "RobotDriveDevRef 2"=w130:T11)  [unwired: 7 in]
      n76 = call-poly <vilib>:"WPI_RobotDriveArcadeDrive.vi"("error in (no error)"=w129, "Y axis value"=0.0, "X axis value"=0.0, "RobotDriveDevRef"=w130) -> ()  [unwired: 5 in, 3 out]
    }
    frame "SHOOTRED" {
      # "SHOOTRED"
      n77 = call <vilib>:"WPI_CANTalonSRX_SetReference.vi"("error in (no error)"=w226, "Feedback Reference"=WPI_CANTalonSRX_APIFeedbackSelect."CTR Magnetic Enc (Relative)", "CAN Talon SRX Ref"=w227) -> ("error out"=w225:errorcluster, "CAN Talon SRX Ref"=w235:T7)  [unwired: 7 in]
      n78 = call <vilib>:"WPI_MotorControlSetOutput.vi"("error in (no error)"=w213, "Output"=0.75, "MotorControlDevRef"=w214) -> ("error out"=w210:errorcluster, "MotorControlDevRef"=w208:T7)  [unwired: 6 in, 1 out]
      n79 = call <vilib>:"WPI_CANTalonSRX_SetPID.vi"("CAN Talon SRX Ref"=w235, "P"=0.0, "I"=0.0, "D"=0.0, "error in (no error)"=w225, "F"=0.01, "I Zone"=0.0, "Ramp Rate"=0.0) -> ("CAN Talon SRX Ref"=w232:T7, "error out"=w224:errorcluster)  [unwired: 6 in]
      n80 = call <vilib>:"WPI_CANTalonSRX_ChangeMode.vi"("error in (no error)"=w224, "Output"=9800.0 ("y"), "Control Mode"=WPI_CANTalonSRX_APIControlMode."Speed", "CAN Talon SRX Ref"=w232) -> ("error out"=w223:errorcluster, "CAN Talon SRX Ref"=w228:T7)  [unwired: 6 in]
      n81 = call <vilib>:"WPI_CANTalonSRX_GetStatus.vi"("error in (no error)"=w223, "CAN Talon SRX Ref"=w228) -> ("error out"=w211:errorcluster, "CAN Talon SRX Ref"=w193:T7)  [unwired: 7 in, 1 out]
      n82 = Merge Errors(w211, w210) -> (w209:errorcluster)
      n83 = call <vilib>:"WPI_RobotDriveDelayAndUpdateSafety.vi"("error in (no error)"=w209, "Delay (s)"=10.0, "RobotDriveDevRef"=w221) -> ("error out"=w192:errorcluster, "RobotDriveDevRef 2"=w222:T11)  [unwired: 7 in]
      n84 = call <vilib>:"WPI_CANTalonSRX_ChangeMode.vi"("error in (no error)"=w192, "Output"=0.0 ("y"), "Control Mode"=WPI_CANTalonSRX_APIControlMode."Speed", "CAN Talon SRX Ref"=w193) -> ("error out"=w194:errorcluster, "CAN Talon SRX Ref"=w195:T7)  [unwired: 6 in]
      n85 = call <vilib>:"WPI_MotorControlSetOutput.vi"("error in (no error)"=w192, "Output"=0.0, "MotorControlDevRef"=w208) -> ("error out"=w190:errorcluster)  [unwired: 6 in, 2 out]
      n86 = call <vilib>:"WPI_CANTalonSRX_GetStatus.vi"("error in (no error)"=w194, "CAN Talon SRX Ref"=w195) -> ("error out"=w191:errorcluster)  [unwired: 7 in, 2 out]
      n87 = Merge Errors(w191, w190) -> (w189:errorcluster)
      n88 = call <vilib>:"WPI_RobotDriveTankDrive.vi"("error in (no error)"=w189, "Right axis value"=0.6 ("Y axis value"), "Left axis value"=0.6, "RobotDriveDevRef"=w222) -> ("error out"=w219:errorcluster, "RobotDriveDevRef"=w220:T11)  [unwired: 5 in, 1 out]
      n89 = call <vilib>:"WPI_RobotDriveDelayAndUpdateSafety.vi"("error in (no error)"=w219, "Delay (s)"=0.25, "RobotDriveDevRef"=w220) -> ("error out"=w201:errorcluster, "RobotDriveDevRef 2"=w200:T11)  [unwired: 7 in]
      n90 = call-poly <vilib>:"WPI_RobotDriveArcadeDrive.vi"("error in (no error)"=w201, "Y axis value"=0.0, "X axis value"=-0.8, "RobotDriveDevRef"=w200) -> ("error out"=w204:errorcluster, "RobotDriveDevRef"=w205:T11)  [unwired: 5 in, 1 out]
      n91 = call <vilib>:"WPI_RobotDriveDelayAndUpdateSafety.vi"("error in (no error)"=w204, "Delay (s)"=0.5, "RobotDriveDevRef"=w205) -> ("error out"=w198:errorcluster, "RobotDriveDevRef 2"=w199:T11)  [unwired: 7 in]
      n92 = call-poly <vilib>:"WPI_RobotDriveArcadeDrive.vi"("error in (no error)"=w198, "Y axis value"=-0.5, "X axis value"=-0.55, "RobotDriveDevRef"=w199) -> ("error out"=w187:errorcluster, "RobotDriveDevRef"=w188:T11)  [unwired: 5 in, 1 out]
      n93 = call <vilib>:"WPI_RobotDriveDelayAndUpdateSafety.vi"("error in (no error)"=w187, "Delay (s)"=1.0, "RobotDriveDevRef"=w188) -> ("error out"=w185:errorcluster, "RobotDriveDevRef 2"=w184:T11)  [unwired: 7 in]
      n94 = call-poly <vilib>:"WPI_RobotDriveArcadeDrive.vi"("error in (no error)"=w185, "Y axis value"=-0.5 ("X axis value"), "RobotDriveDevRef"=w184) -> ("error out"=w179:errorcluster, "RobotDriveDevRef"=w180:T11)  [unwired: 6 in, 1 out]
      n95 = call <vilib>:"WPI_RobotDriveDelayAndUpdateSafety.vi"("error in (no error)"=w179, "Delay (s)"=2.0, "RobotDriveDevRef"=w180) -> ("error out"=w176:errorcluster, "RobotDriveDevRef 2"=w177:T11)  [unwired: 7 in]
      n96 = call-poly <vilib>:"WPI_RobotDriveArcadeDrive.vi"("error in (no error)"=w176, "Y axis value"=0.0, "X axis value"=0.0, "RobotDriveDevRef"=w177) -> ()  [unwired: 5 in, 3 out]
    }
    frame "NEW" {
      n97 = while {
        tunnel: w261 -> [w353]
        tunnel: w260 -> [w352]
        tunnel: [w346] -> w262
        tunnel: [w345] -> w263
        tunnel: w259 -> [w344]
        tunnel: w258 -> [w338]
        tunnel: [w334] -> w257
        tunnel: [w333] -> w256
        tunnel: w247 -> [w332]
        tunnel: [w332] -> w246
        stop <- w335 stop-if-true
        n98 = call <vilib>:"WPI_EncoderGet.vi"("EncoderDevRef"=w344) -> ("Distance"=w343:dbl, "EncoderDevRef"=w334:T3)  [unwired: 5 in, 4 out]
        n99 = call <vilib>:"WPI_EncoderGet.vi"("EncoderDevRef"=w353) -> ("Distance"=w351:dbl, "EncoderDevRef"=w345:T3)  [unwired: 5 in, 4 out]
        n100 = Greater?(x=w343, y=4.0) -> (0:w336:bool)
        n101 = Greater?(x=w351, y=4.0) -> (0:w337:bool)
        n102 = Select(t=0.0, s=w336, f=-0.3) -> (s? t:f=w339:dbl)
        n103 = Select(t=0.0, s=w337, f=-0.3) -> (s? t:f=w347:dbl)
        n104 = And(x=w337, y=w336) -> (x .and. y?=w335:bool)
        n105 = call <vilib>:"WPI_MotorControlSetOutput.vi"("Output"=w339, "MotorControlDevRef"=w338) -> ("MotorControlDevRef"=w333:T7)  [unwired: 7 in, 2 out]
        n106 = call <vilib>:"WPI_MotorControlSetOutput.vi"("Output"=w347, "MotorControlDevRef"=w352) -> ("MotorControlDevRef"=w346:T7)  [unwired: 7 in, 2 out]
      }
      n107 = while {
        tunnel: [w328] -> w255
        tunnel: [w327] -> w254
        tunnel: w263 -> [w326]
        tunnel: w262 -> [w325]
        tunnel: w257 -> [w321]
        tunnel: w256 -> [w320]
        tunnel: [w321] -> w253
        tunnel: [w320] -> w252
        tunnel: w246 -> [w319]
        tunnel: [w319] -> w245
        stop <- w322 continue-if-true
        n108 = call <vilib>:"WPI_EncoderGet.vi"("EncoderDevRef"=w326) -> ("Distance"=w324:dbl, "EncoderDevRef"=w328:T3)  [unwired: 5 in, 4 out]
        n109 = Greater?(x=4.0 ("y"), y=w324) -> (0:w322:bool)
        n110 = Select(t=0.3, s=w322, f=0.0 ("Output")) -> (s? t:f=w329:dbl)
        n111 = call <vilib>:"WPI_MotorControlSetOutput.vi"("Output"=w329, "MotorControlDevRef"=w325) -> ("MotorControlDevRef"=w327:T7)  [unwired: 7 in, 2 out]
      }
      n112 = while {
        tunnel: w255 -> [w318]
        tunnel: w254 -> [w317]
        tunnel: [w311] -> w248
        tunnel: [w310] -> w249
        tunnel: w253 -> [w309]
        tunnel: w252 -> [w303]
        tunnel: [w299] -> w250
        tunnel: [w298] -> w251
        tunnel: w245 -> [w297]
        tunnel: [w297] -> w244
        stop <- w300 stop-if-true
        n113 = call <vilib>:"WPI_EncoderGet.vi"("EncoderDevRef"=w309) -> ("Distance"=w308:dbl, "EncoderDevRef"=w299:T3)  [unwired: 5 in, 4 out]
        n114 = call <vilib>:"WPI_EncoderGet.vi"("EncoderDevRef"=w318) -> ("Distance"=w316:dbl, "EncoderDevRef"=w310:T3)  [unwired: 5 in, 4 out]
        n115 = Greater?(x=w308, y=4.0) -> (0:w301:bool)
        n116 = Greater?(x=w316, y=4.0) -> (0:w302:bool)
        n117 = Select(t=0.0, s=w301, f=-0.3) -> (s? t:f=w304:dbl)
        n118 = Select(t=0.0, s=w302, f=-0.3) -> (s? t:f=w312:dbl)
        n119 = And(x=w302, y=w301) -> (x .and. y?=w300:bool)
        n120 = call <vilib>:"WPI_MotorControlSetOutput.vi"("Output"=w304, "MotorControlDevRef"=w303) -> ("MotorControlDevRef"=w298:T7)  [unwired: 7 in, 2 out]
        n121 = call <vilib>:"WPI_MotorControlSetOutput.vi"("Output"=w312, "MotorControlDevRef"=w317) -> ("MotorControlDevRef"=w311:T7)  [unwired: 7 in, 2 out]
      }
      n122 = while {
        tunnel: w251 -> [w288]
        tunnel: w250 -> [w287]
        tunnel: w249 -> [w285]
        tunnel: w248 -> [w286]
        tunnel: w244 -> [w296]
        tunnel: [w288] -> w243
        tunnel: [w287] -> w242
        tunnel: [w286] -> w241
        tunnel: [w285] -> w240
        stop <- w289 stop-if-true
        n123 = global read "Robot Global Data.vi" "LOWER LIMIT"() -> (w292:bool)
        n124 = Select(t=0.0, s=w292, f=-0.5) -> (s? t:f=w293:dbl)
        n125 = call <vilib>:"WPI_MotorControlSetOutput.vi"("Output"=w293, "MotorControlDevRef"=w296) -> ("Motor Output"=w291:dbl)  [unwired: 7 in, 2 out]
        n126 = Equal?(x=w291, y=0.0) -> (x = y?=w289:bool)
      }
      n127 = while {
        tunnel: [w279] -> _
        tunnel: [w278] -> _
        tunnel: [w269] -> _
        tunnel: [w268] -> _
        tunnel: w243 -> [w267]
        tunnel: w242 -> [w266]
        tunnel: w241 -> [w265]
        tunnel: w240 -> [w264]
        stop <- w270 stop-if-true
        n128 = call <vilib>:"WPI_EncoderGet.vi"("EncoderDevRef"=w266) -> ("Distance"=w277:dbl, "EncoderDevRef"=w269:T3)  [unwired: 5 in, 4 out]
        n129 = call <vilib>:"WPI_EncoderGet.vi"("EncoderDevRef"=w264) -> ("Distance"=w284:dbl, "EncoderDevRef"=w278:T3)  [unwired: 5 in, 4 out]
        n130 = Greater?(x=w277, y=0.0) -> (0:w271:bool)
        n131 = Greater?(x=w284, y=0.0) -> (0:w272:bool)
        n132 = Select(t=-0.3, s=w271, f=0.0) -> (s? t:f=w273:dbl)
        n133 = Select(t=-0.3, s=w272, f=0.0) -> (s? t:f=w280:dbl)
        n134 = And(x=w272, y=w271) -> (x .and. y?=w270:bool)
        n135 = call <vilib>:"WPI_MotorControlSetOutput.vi"("Output"=w273, "MotorControlDevRef"=w267) -> ("MotorControlDevRef"=w268:T7)  [unwired: 7 in, 2 out]
        n136 = call <vilib>:"WPI_MotorControlSetOutput.vi"("Output"=w280, "MotorControlDevRef"=w265) -> ("MotorControlDevRef"=w279:T7)  [unwired: 7 in, 2 out]
      }
    }
    frame "RANDOM" {
      n137 = while {
        tunnel: w360 -> [w400]
        tunnel: w361 -> [w399]
        tunnel: [w395] -> w354
        tunnel: [w394] -> w355
        tunnel: w359 -> [w393]
        tunnel: w358 -> [w389]
        tunnel: [w388] -> w356
        tunnel: [w387] -> w357
        stop <- w383 continue-if-true
        n138 = call <vilib>:"WPI_EncoderGet.vi"("EncoderDevRef"=w393) -> ("EncoderDevRef"=w388:T3)  [unwired: 5 in, 5 out]
        n139 = call <vilib>:"WPI_EncoderGet.vi"("EncoderDevRef"=w400) -> ("Distance"=w384:dbl, "EncoderDevRef"=w394:T3)  [unwired: 5 in, 4 out]
        "Distance" <- w384
        n140 = In Range and Coerce(upper limit=7.4, x=w384, lower limit=0.0) -> (In Range?=w383:bool)  [unwired: 1 out]
        n141 = Select(t=0.3, s=w383, f=0.0) -> (s? t:f=w390:dbl)
        n142 = Select(t=0.3, s=w383, f=0.0) -> (s? t:f=w396:dbl)
        n143 = call <vilib>:"WPI_MotorControlSetOutput.vi"("Output"=w390, "MotorControlDevRef"=w389) -> ("MotorControlDevRef"=w387:T7)  [unwired: 7 in, 2 out]
        n144 = call <vilib>:"WPI_MotorControlSetOutput.vi"("Output"=w396, "MotorControlDevRef"=w399) -> ("MotorControlDevRef"=w395:T7)  [unwired: 7 in, 2 out]
      }
      n145 = while {
        tunnel: w355 -> [w382]
        tunnel: w354 -> [w381]
        tunnel: [w375] -> _
        tunnel: [w374] -> _
        tunnel: w356 -> [w373]
        tunnel: w357 -> [w367]
        tunnel: [w363] -> _
        tunnel: [w362] -> _
        stop <- w364 stop-if-true
        n146 = call <vilib>:"WPI_EncoderGet.vi"("EncoderDevRef"=w373) -> ("Distance"=w372:dbl, "EncoderDevRef"=w363:T3)  [unwired: 5 in, 4 out]
        n147 = call <vilib>:"WPI_EncoderGet.vi"("EncoderDevRef"=w382) -> ("Distance"=w380:dbl, "EncoderDevRef"=w374:T3)  [unwired: 5 in, 4 out]
        n148 = Greater?(x=w372, y=0.0) -> (0:w365:bool)
        n149 = Greater?(x=w380, y=0.0) -> (0:w366:bool)
        n150 = Select(t=-0.3, s=w365, f=0.0) -> (s? t:f=w368:dbl)
        n151 = Select(t=-0.3, s=w366, f=0.0) -> (s? t:f=w376:dbl)
        n152 = And(x=w366, y=w365) -> (x .and. y?=w364:bool)
        n153 = call <vilib>:"WPI_MotorControlSetOutput.vi"("Output"=w368, "MotorControlDevRef"=w367) -> ("MotorControlDevRef"=w362:T7)  [unwired: 7 in, 2 out]
        n154 = call <vilib>:"WPI_MotorControlSetOutput.vi"("Output"=w376, "MotorControlDevRef"=w381) -> ("MotorControlDevRef"=w375:T7)  [unwired: 7 in, 2 out]
      }
    }
    frame "MIDDLE" {
      n155 = call-poly <vilib>:"WPI_RobotDriveArcadeDrive.vi"("error in (no error)"=w430, "Y axis value"=0.45, "RobotDriveDevRef"=w431) -> ("error out"=w427:errorcluster, "RobotDriveDevRef"=w428:T11)  [unwired: 6 in, 1 out]
      n156 = call <vilib>:"WPI_RobotDriveDelayAndUpdateSafety.vi"("error in (no error)"=w427, "Delay (s)"=2.0, "RobotDriveDevRef"=w428) -> ("error out"=w425:errorcluster, "RobotDriveDevRef 2"=w424:T11)  [unwired: 7 in]
      n157 = call-poly <vilib>:"WPI_RobotDriveArcadeDrive.vi"("error in (no error)"=w425, "Y axis value"=0.0, "RobotDriveDevRef"=w424) -> ("error out"=w421:errorcluster, "RobotDriveDevRef"=w422:T11)  [unwired: 6 in, 1 out]
      n158 = call <vilib>:"WPI_RobotDriveDelayAndUpdateSafety.vi"("error in (no error)"=w421, "Delay (s)"=0.5, "RobotDriveDevRef"=w422) -> ("error out"=w419:errorcluster, "RobotDriveDevRef 2"=w417:T11)  [unwired: 7 in]
      n159 = call <vilib>:"WPI_MotorControlSetOutput.vi"("error in (no error)"=w419, "Output"=-0.7, "MotorControlDevRef"=w418) -> ("error out"=w416:errorcluster, "MotorControlDevRef"=w412:T7)  [unwired: 6 in, 1 out]
      n160 = call <vilib>:"WPI_RobotDriveDelayAndUpdateSafety.vi"("error in (no error)"=w416, "Delay (s)"=1.5, "RobotDriveDevRef"=w417) -> ("error out"=w413:errorcluster, "RobotDriveDevRef 2"=w410:T11)  [unwired: 7 in]
      n161 = call <vilib>:"WPI_MotorControlSetOutput.vi"("error in (no error)"=w413, "Output"=0.0, "MotorControlDevRef"=w412) -> ("error out"=w409:errorcluster)  [unwired: 6 in, 2 out]
      n162 = call-poly <vilib>:"WPI_RobotDriveArcadeDrive.vi"("error in (no error)"=w409, "Y axis value"=-0.4, "RobotDriveDevRef"=w410) -> ("error out"=w406:errorcluster, "RobotDriveDevRef"=w407:T11)  [unwired: 6 in, 1 out]
      n163 = call <vilib>:"WPI_RobotDriveDelayAndUpdateSafety.vi"("error in (no error)"=w406, "Delay (s)"=2.0, "RobotDriveDevRef"=w407) -> ("error out"=w403:errorcluster, "RobotDriveDevRef 2"=w404:T11)  [unwired: 7 in]
      n164 = call-poly <vilib>:"WPI_RobotDriveArcadeDrive.vi"("error in (no error)"=w403, "Y axis value"=0.0, "X axis value"=0.0, "RobotDriveDevRef"=w404) -> ()  [unwired: 5 in, 3 out]
    }
    frame "RIGHTSIDE" {
      # "RIGHTSIDE"
      n165 = call-poly <vilib>:"WPI_RobotDriveArcadeDrive.vi"("error in (no error)"=w433, "Y axis value"=0.59, "RobotDriveDevRef"=w434) -> ("error out"=w473:errorcluster, "RobotDriveDevRef"=w474:T11)  [unwired: 6 in, 1 out]
      n166 = call <vilib>:"WPI_RobotDriveDelayAndUpdateSafety.vi"("error in (no error)"=w473, "Delay (s)"=1.8, "RobotDriveDevRef"=w474) -> ("error out"=w469:errorcluster, "RobotDriveDevRef 2"=w470:T11)  [unwired: 7 in]
      n167 = call-poly <vilib>:"WPI_RobotDriveArcadeDrive.vi"("error in (no error)"=w469, "X axis value"=0.36, "RobotDriveDevRef"=w470) -> ("error out"=w466:errorcluster, "RobotDriveDevRef"=w467:T11)  [unwired: 6 in, 1 out]
      n168 = call <vilib>:"WPI_RobotDriveDelayAndUpdateSafety.vi"("error in (no error)"=w466, "Delay (s)"=1.0, "RobotDriveDevRef"=w467) -> ("error out"=w463:errorcluster, "RobotDriveDevRef 2"=w464:T11)  [unwired: 7 in]
      n169 = call-poly <vilib>:"WPI_RobotDriveArcadeDrive.vi"("error in (no error)"=w463, "Y axis value"=0.5, "RobotDriveDevRef"=w464) -> ("error out"=w460:errorcluster, "RobotDriveDevRef"=w461:T11)  [unwired: 6 in, 1 out]
      n170 = call <vilib>:"WPI_RobotDriveDelayAndUpdateSafety.vi"("error in (no error)"=w460, "Delay (s)"=2.3, "RobotDriveDevRef"=w461) -> ("error out"=w457:errorcluster, "RobotDriveDevRef 2"=w458:T11)  [unwired: 7 in]
      n171 = call-poly <vilib>:"WPI_RobotDriveArcadeDrive.vi"("error in (no error)"=w457, "Y axis value"=0.0, "RobotDriveDevRef"=w458) -> ("error out"=w454:errorcluster, "RobotDriveDevRef"=w455:T11)  [unwired: 6 in, 1 out]
      n172 = call <vilib>:"WPI_RobotDriveDelayAndUpdateSafety.vi"("error in (no error)"=w454, "Delay (s)"=0.5, "RobotDriveDevRef"=w455) -> ("error out"=w452:errorcluster, "RobotDriveDevRef 2"=w450:T11)  [unwired: 7 in]
      n173 = call <vilib>:"WPI_MotorControlSetOutput.vi"("error in (no error)"=w452, "Output"=-0.7, "MotorControlDevRef"=w432) -> ("error out"=w449:errorcluster, "MotorControlDevRef"=w438:T7)  [unwired: 6 in, 1 out]
      n174 = call <vilib>:"WPI_RobotDriveDelayAndUpdateSafety.vi"("error in (no error)"=w449, "Delay (s)"=1.5, "RobotDriveDevRef"=w450) -> ("error out"=w437:errorcluster, "RobotDriveDevRef 2"=w447:T11)  [unwired: 7 in]
      n175 = call <vilib>:"WPI_MotorControlSetOutput.vi"("error in (no error)"=w437, "Output"=0.0, "MotorControlDevRef"=w438) -> ("error out"=w435:errorcluster)  [unwired: 6 in, 2 out]
      n176 = call-poly <vilib>:"WPI_RobotDriveArcadeDrive.vi"("error in (no error)"=w435, "Y axis value"=-0.4, "RobotDriveDevRef"=w447) -> ("error out"=w444:errorcluster, "RobotDriveDevRef"=w445:T11)  [unwired: 6 in, 1 out]
      n177 = call <vilib>:"WPI_RobotDriveDelayAndUpdateSafety.vi"("error in (no error)"=w444, "Delay (s)"=2.0, "RobotDriveDevRef"=w445) -> ("error out"=w442:errorcluster, "RobotDriveDevRef 2"=w441:T11)  [unwired: 7 in]
      n178 = call-poly <vilib>:"WPI_RobotDriveArcadeDrive.vi"("error in (no error)"=w442, "Y axis value"=0.0, "X axis value"=0.0, "RobotDriveDevRef"=w441) -> ()  [unwired: 5 in, 3 out]
    }
    frame "LEFTSIDE" {
      n179 = call-poly <vilib>:"WPI_RobotDriveArcadeDrive.vi"("error in (no error)"=w516, "Y axis value"=0.6, "RobotDriveDevRef"=w517) -> ("error out"=w514:errorcluster, "RobotDriveDevRef"=w515:T11)  [unwired: 6 in, 1 out]
      n180 = call <vilib>:"WPI_RobotDriveDelayAndUpdateSafety.vi"("error in (no error)"=w514, "Delay (s)"=2.0, "RobotDriveDevRef"=w515) -> ("error out"=w510:errorcluster, "RobotDriveDevRef 2"=w511:T11)  [unwired: 7 in]
      n181 = call-poly <vilib>:"WPI_RobotDriveArcadeDrive.vi"("error in (no error)"=w510, "X axis value"=-0.45, "RobotDriveDevRef"=w511) -> ("error out"=w507:errorcluster, "RobotDriveDevRef"=w508:T11)  [unwired: 6 in, 1 out]
      n182 = call <vilib>:"WPI_RobotDriveDelayAndUpdateSafety.vi"("error in (no error)"=w507, "Delay (s)"=1.0, "RobotDriveDevRef"=w508) -> ("error out"=w504:errorcluster, "RobotDriveDevRef 2"=w505:T11)  [unwired: 7 in]
      n183 = call-poly <vilib>:"WPI_RobotDriveArcadeDrive.vi"("error in (no error)"=w504, "Y axis value"=0.52, "RobotDriveDevRef"=w505) -> ("error out"=w501:errorcluster, "RobotDriveDevRef"=w502:T11)  [unwired: 6 in, 1 out]
      n184 = call <vilib>:"WPI_RobotDriveDelayAndUpdateSafety.vi"("error in (no error)"=w501, "Delay (s)"=2.25, "RobotDriveDevRef"=w502) -> ("error out"=w498:errorcluster, "RobotDriveDevRef 2"=w499:T11)  [unwired: 7 in]
      n185 = call-poly <vilib>:"WPI_RobotDriveArcadeDrive.vi"("error in (no error)"=w498, "Y axis value"=0.0, "RobotDriveDevRef"=w499) -> ("error out"=w495:errorcluster, "RobotDriveDevRef"=w496:T11)  [unwired: 6 in, 1 out]
      n186 = call <vilib>:"WPI_RobotDriveDelayAndUpdateSafety.vi"("error in (no error)"=w495, "Delay (s)"=0.5, "RobotDriveDevRef"=w496) -> ("error out"=w492:errorcluster, "RobotDriveDevRef 2"=w490:T11)  [unwired: 7 in]
      n187 = call <vilib>:"WPI_MotorControlSetOutput.vi"("error in (no error)"=w492, "Output"=-0.7, "MotorControlDevRef"=w493) -> ("error out"=w489:errorcluster, "MotorControlDevRef"=w478:T7)  [unwired: 6 in, 1 out]
      n188 = call <vilib>:"WPI_RobotDriveDelayAndUpdateSafety.vi"("error in (no error)"=w489, "Delay (s)"=1.5, "RobotDriveDevRef"=w490) -> ("error out"=w477:errorcluster, "RobotDriveDevRef 2"=w487:T11)  [unwired: 7 in]
      n189 = call <vilib>:"WPI_MotorControlSetOutput.vi"("error in (no error)"=w477, "Output"=0.0, "MotorControlDevRef"=w478) -> ("error out"=w475:errorcluster)  [unwired: 6 in, 2 out]
      n190 = call-poly <vilib>:"WPI_RobotDriveArcadeDrive.vi"("error in (no error)"=w475, "Y axis value"=-0.4, "RobotDriveDevRef"=w487) -> ("error out"=w484:errorcluster, "RobotDriveDevRef"=w485:T11)  [unwired: 6 in, 1 out]
      n191 = call <vilib>:"WPI_RobotDriveDelayAndUpdateSafety.vi"("error in (no error)"=w484, "Delay (s)"=2.0, "RobotDriveDevRef"=w485) -> ("error out"=w482:errorcluster, "RobotDriveDevRef 2"=w481:T11)  [unwired: 7 in]
      n192 = call-poly <vilib>:"WPI_RobotDriveArcadeDrive.vi"("error in (no error)"=w482, "Y axis value"=0.0, "X axis value"=0.0, "RobotDriveDevRef"=w481) -> ()  [unwired: 5 in, 3 out]
    }
    frame "Forward" {
      n193 = call-poly <vilib>:"WPI_RobotDriveArcadeDrive.vi"("error in (no error)"=w522, "Y axis value"=0.55, "RobotDriveDevRef"=w523) -> ("error out"=w518:errorcluster, "RobotDriveDevRef"=w520:T11)  [unwired: 6 in, 1 out]
      n194 = call <vilib>:"WPI_RobotDriveDelayAndUpdateSafety.vi"("error in (no error)"=w518, "Delay (s)"=2.8, "RobotDriveDevRef"=w520) -> ()  [unwired: 7 in, 2 out]
    }
    frame "GEAR DROP" {
      n195 = call-poly <vilib>:"WPI_RobotDriveArcadeDrive.vi"("error in (no error)"=w547, "Y axis value"=0.45, "RobotDriveDevRef"=w548) -> ("error out"=w544:errorcluster, "RobotDriveDevRef"=w545:T11)  [unwired: 6 in, 1 out]
      n196 = call <vilib>:"WPI_RobotDriveDelayAndUpdateSafety.vi"("error in (no error)"=w544, "Delay (s)"=2.4, "RobotDriveDevRef"=w545) -> ("error out"=w542:errorcluster, "RobotDriveDevRef 2"=w541:T11)  [unwired: 7 in]
      n197 = call-poly <vilib>:"WPI_RobotDriveArcadeDrive.vi"("error in (no error)"=w542, "Y axis value"=0.0, "RobotDriveDevRef"=w541) -> ("error out"=w538:errorcluster, "RobotDriveDevRef"=w539:T11)  [unwired: 6 in, 1 out]
      n198 = call <vilib>:"WPI_RobotDriveDelayAndUpdateSafety.vi"("error in (no error)"=w538, "Delay (s)"=0.5, "RobotDriveDevRef"=w539) -> ("error out"=w531:errorcluster, "RobotDriveDevRef 2"=w530:T11)  [unwired: 7 in]
      n199 = while {
        tunnel: w531 -> [w560]
        tunnel: [w557] -> w529
        tunnel: w528 -> [w556]
        tunnel: [w555] -> w527
        stop <- w558 stop-if-true
        n200 = global read "Robot Global Data.vi" "LOWER LIMIT"() -> (w558:bool)
        n201 = call <vilib>:"WPI_MotorControlSetOutput.vi"("error in (no error)"=w560, "Output"=-0.6 ("f"), "MotorControlDevRef"=w556) -> ("error out"=w557:errorcluster, "MotorControlDevRef"=w555:T7)  [unwired: 6 in, 1 out]
      }
      n202 = call-poly <vilib>:"WPI_RobotDriveArcadeDrive.vi"("error in (no error)"=w529, "Y axis value"=-0.4, "RobotDriveDevRef"=w530) -> ("error out"=w535:errorcluster, "RobotDriveDevRef"=w534:T11)  [unwired: 6 in, 1 out]
      n203 = call <vilib>:"WPI_RobotDriveDelayAndUpdateSafety.vi"("error in (no error)"=w535, "Delay (s)"=1.5, "RobotDriveDevRef"=w534) -> ("error out"=w526:errorcluster)  [unwired: 7 in, 1 out]
      n204 = while {
        tunnel: w527 -> [w553]
        tunnel: w526 -> [w551]
        tunnel: [w550] -> w525
        tunnel: [w549] -> w524
        stop <- w554 stop-if-true
        n205 = call <vilib>:"WPI_MotorControlSetOutput.vi"("error in (no error)"=w551, "Output"=0.6, "MotorControlDevRef"=w553) -> ("error out"=w549:errorcluster, "MotorControlDevRef"=w550:T7)  [unwired: 6 in, 1 out]
        n206 = global read "Robot Global Data.vi" "UPPER LIMIT"() -> (w554:bool)
      }
      n207 = call <vilib>:"WPI_MotorControlSetOutput.vi"("error in (no error)"=w524, "Output"=0.0, "MotorControlDevRef"=w525) -> ()  [unwired: 6 in, 3 out]
    }
  }
